vi "Collision Detection top level.vi"(0 "Model rotation (degrees)":sgl, 1 "Model rotation axis (unit vector)":sgl[](array[numeric])=[0.0, 0.0, 1.0], 3 "Model rotation axis coordinates (absolute, mm)":sgl[](array[numeric])=[0.0, 0.0, 0.0], 4 "Collision mode":T1=enum."Traverse - All", 5 "Get minimum separation within look-out sphere":bool, 6 "Traverse position (absolute, mm)":sgl[](array[numeric])=[0.0, 0.0, 0.0], 7 "3D graphics output":bool, 9 "Visualisation only (no collision detection)":bool, 10 "Traverse name":string="EnFlo_Trav1", 11 "Extrusion mode":bool, 12 "Rig geometry directory path":path=path "C:/EnFlo_Data_Local/Preferences/Rig_Setups/EnFlo_Tunnel/All_Users/Collision_detection", 13 "Traverse extruded position":sgl[](array[numeric])=[0.0, 0.0, 0.0]) -> (14 "Collision":bool, 15 "Collision point(s)":sgl[][](array[numeric]), 16 "Traverse collision part":cluster{"X":bool, "XY":bool, "XYZ":bool}, 17 "Minimum separation":sgl, 18 "Minimum separation vector (from trav.)":sgl[](array[numeric]), 19 "Error out":errorcluster)   [LabVIEW 2016]
uses:
  Collision Mode.ctl
  Typedefs/Triangle.ctl
  <vilib>/Utility/miscctls.llb/LVRGBAColorTypeDef.ctl
  Convex Hull/Subroutines/Coincident points test.vi
  Subroutines/Cross product 3D.vi
  Subroutines/Unit vector.vi
  Collision Detection global.vi
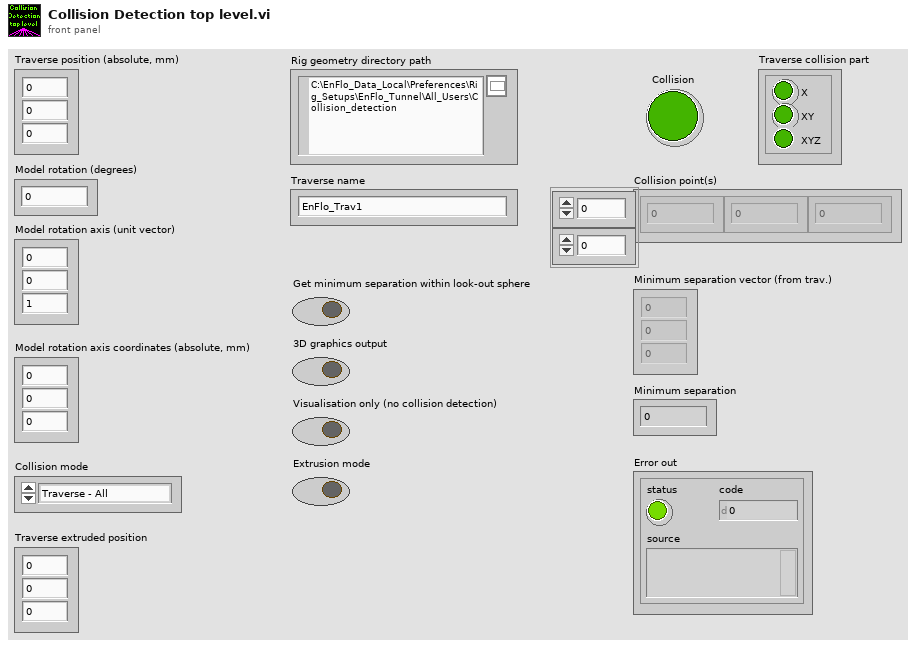
[diagram p1: front panel]
types:
  T1 = typedef "Collision Mode.ctl" = enum16{"Traverse - Tunnel", "Traverse - Model", "Traverse - Fixed objects", "Traverse - Traverse", "Traverse - All"}
  T2 = typedef "Traverse active parts.ctl" = enum16{"XYZ", "XY and XYZ", "X and XY and XYZ"}
  T3 = cluster{"Red":sgl, "Green":sgl, "Blue":sgl, "Alpha":sgl}
  T4 = typedef "LVRGBAColorTypeDef.ctl" = cluster{"Red":sgl, "Green":sgl, "Blue":sgl, "Alpha":sgl}
  T5 = typedef "TreeNodeBox.ctl" = cluster{"Face 0":T6, "Face 1":T6, "Face 2":T6, "Face 3":T6, "Face 4":T6, "Face 5":T6, "Level":i32, "Pmax":sgl[], "Pmin":sgl[], "Parent":i32, "Child 1":i32, "Child 2":i32, "Child 3":i32, "Child 4":i32, "Child 5":i32, "Child 6":i32, "Child 7":i32, "Child 8":i32, "Triangles":i32[], "is leaf node":bool}
  T6 = typedef "Quad.ctl" = cluster{"V0":sgl[], "V1":sgl[], "V2":sgl[], "V3":sgl[], "E0":sgl[], "E1":sgl[], "E2":sgl[], "E3":sgl[], "n^":sgl[], "Plane":T7}
  T7 = typedef "Quadplane enum.ctl" = enum8{"XY", "XZ", "YZ", "-XY", "-XZ", "-YZ"}
  T8 = typedef "Triangle.ctl" = cluster{"V0":sgl[], "V1":sgl[], "V2":sgl[], "E0":sgl[], "E1":sgl[], "E2":sgl[], "n^":sgl[], "nE0^":sgl[], "nE1^":sgl[], "nE2^":sgl[]}
  T9 = typedef "Sphere.ctl" = cluster{"Centre":sgl[], "Radius":sgl}
  T10 = typedef "Triangle, indexed.ctl" = cluster{"V0":sgl[], "V1":sgl[], "V2":sgl[], "n^":sgl[], "i0":i32, "i1":i32, "i2":i32}
  T11 = enum16{"Inherit Value", "Points", "Wireframe", "Polygons"}
  T12 = typedef "LV3DPointTypeDef.ctl" = cluster{"X":sgl, "Y":sgl, "Z":sgl}
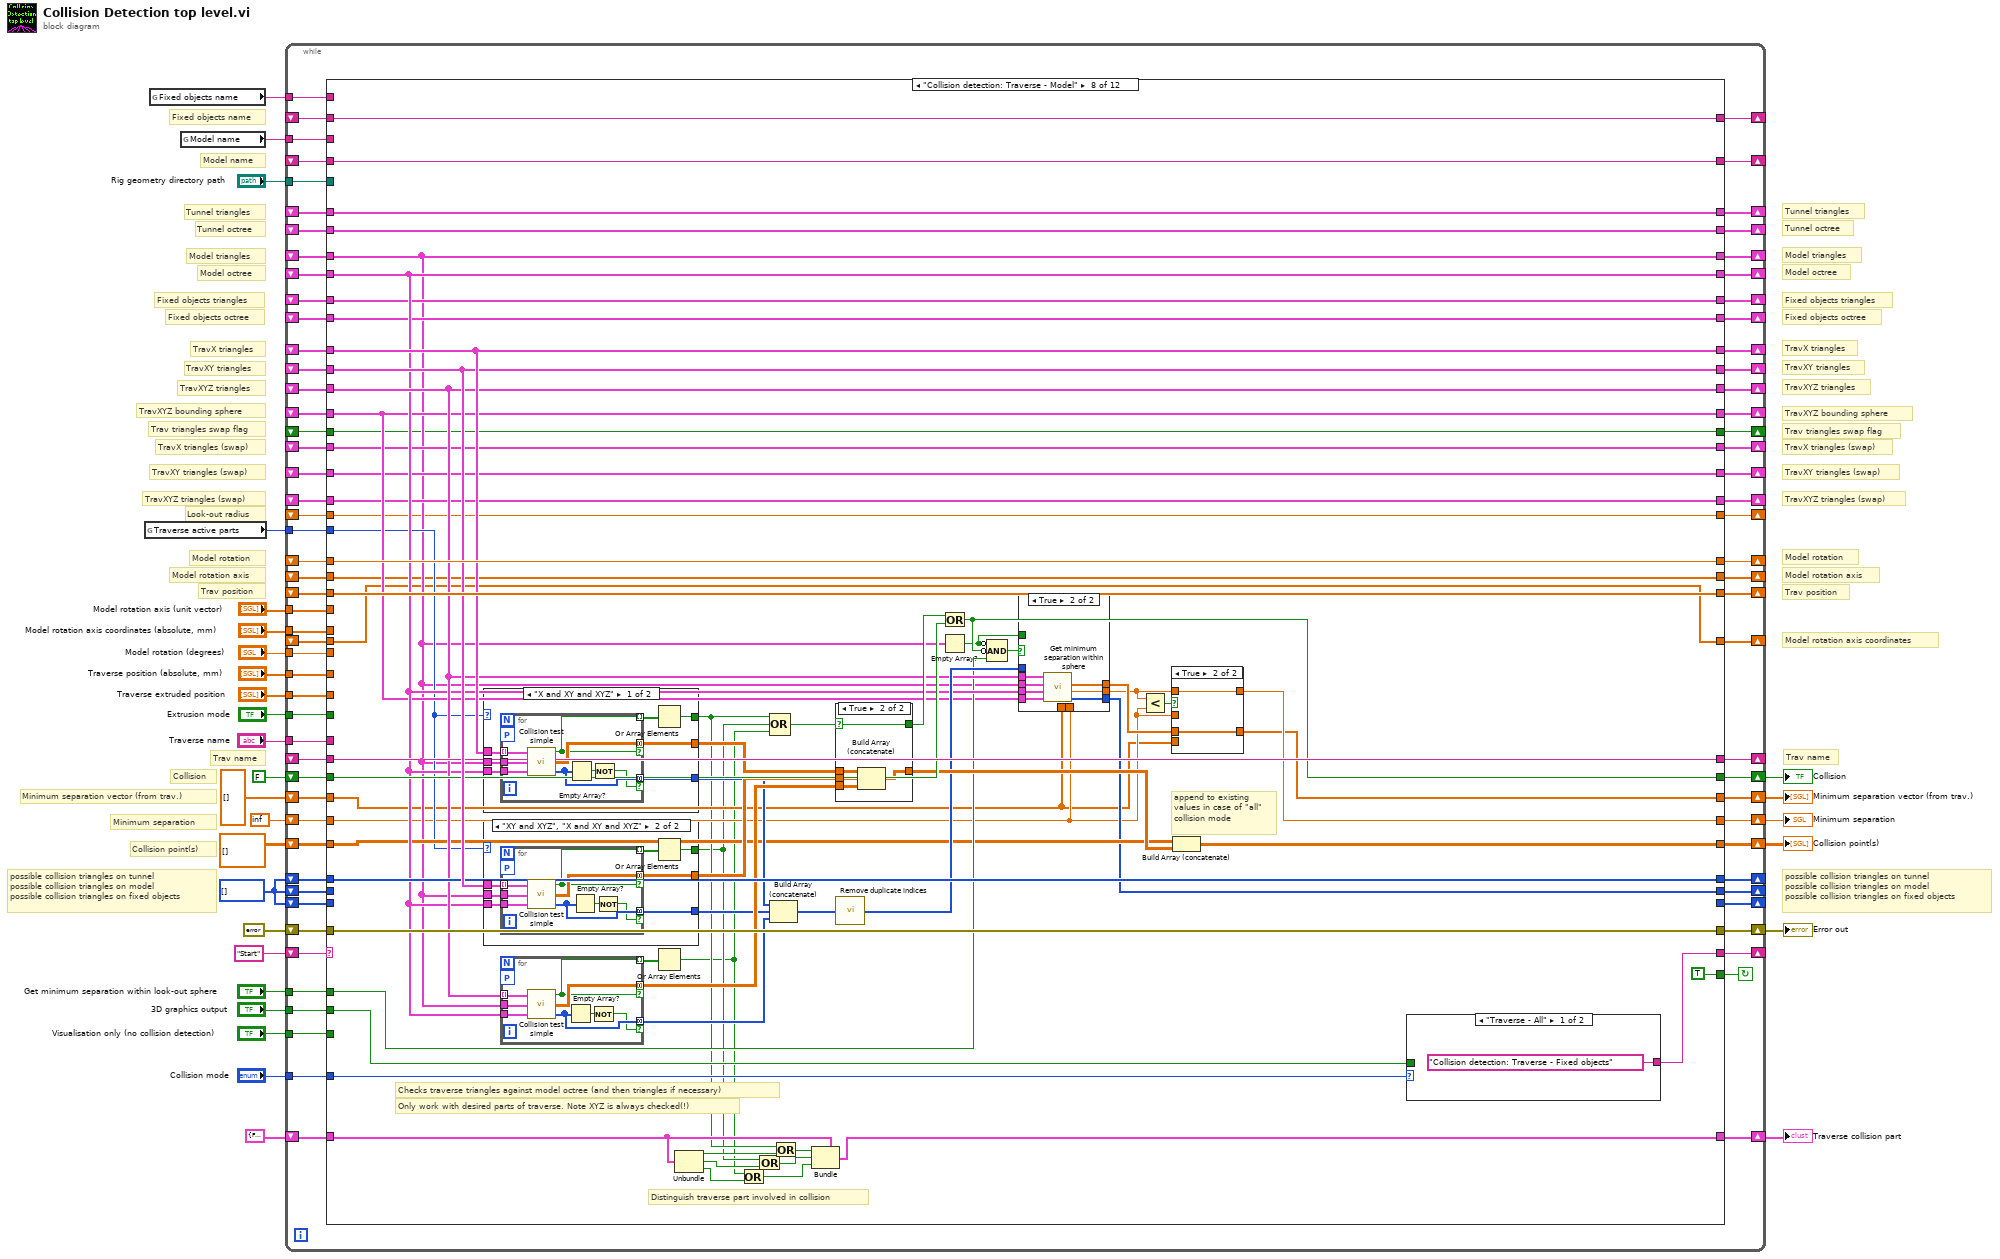
[diagram p0: block diagram]
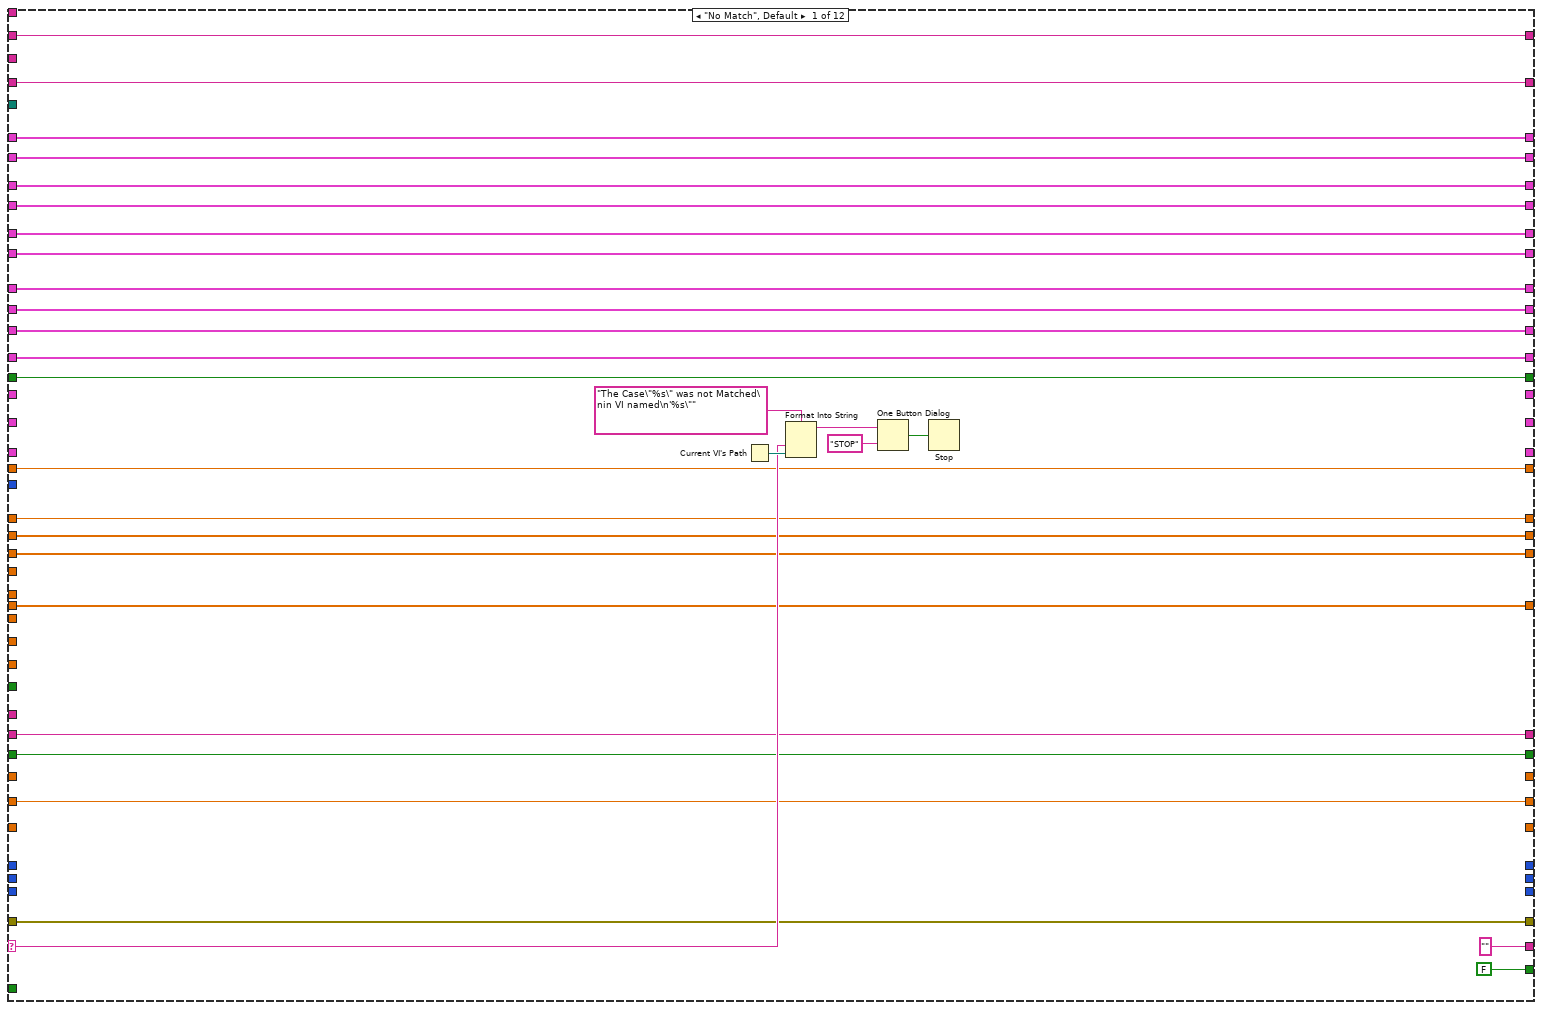
[diagram p2: hidden frame]
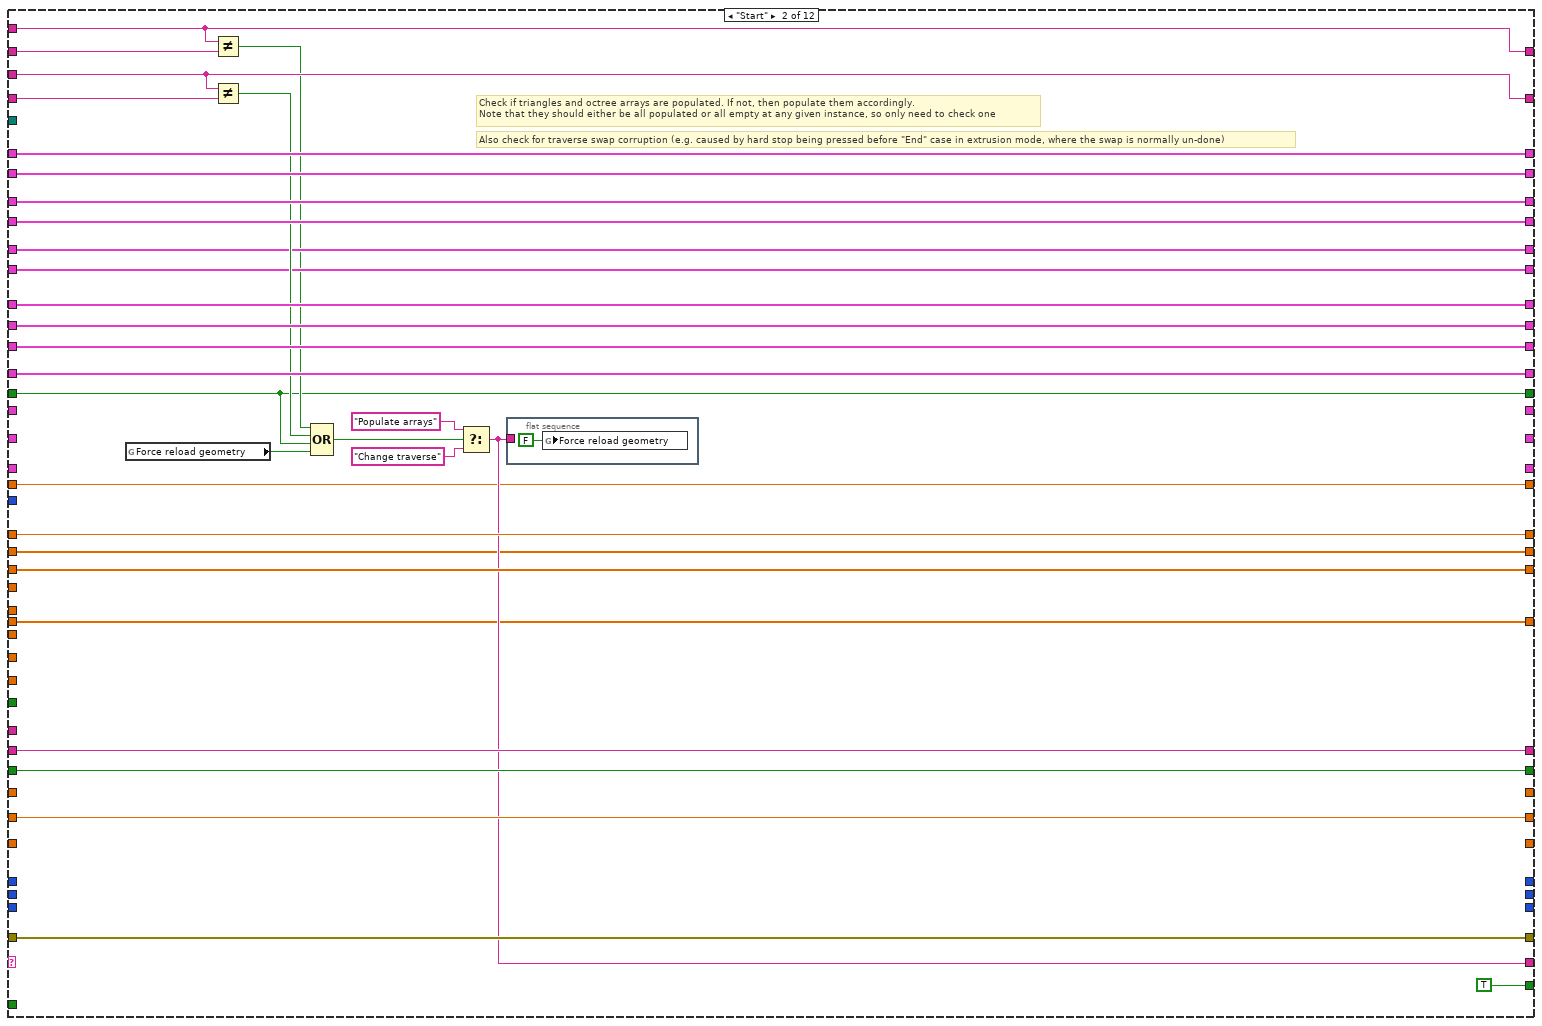
[diagram p3: hidden frame]
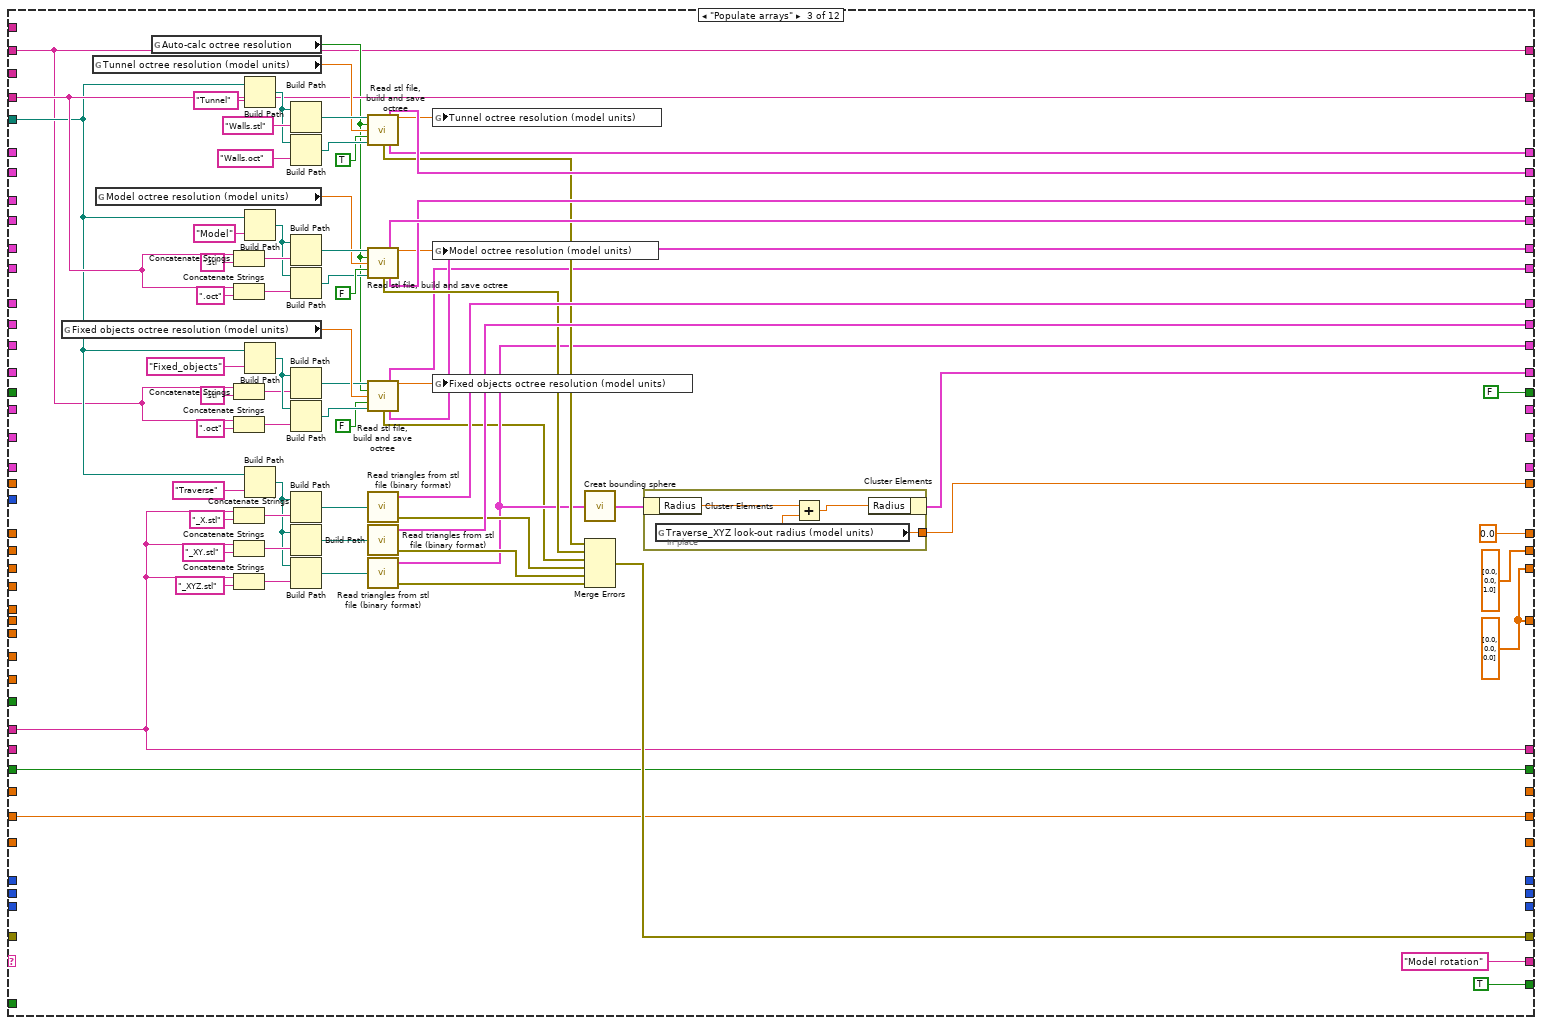
[diagram p4: hidden frame]
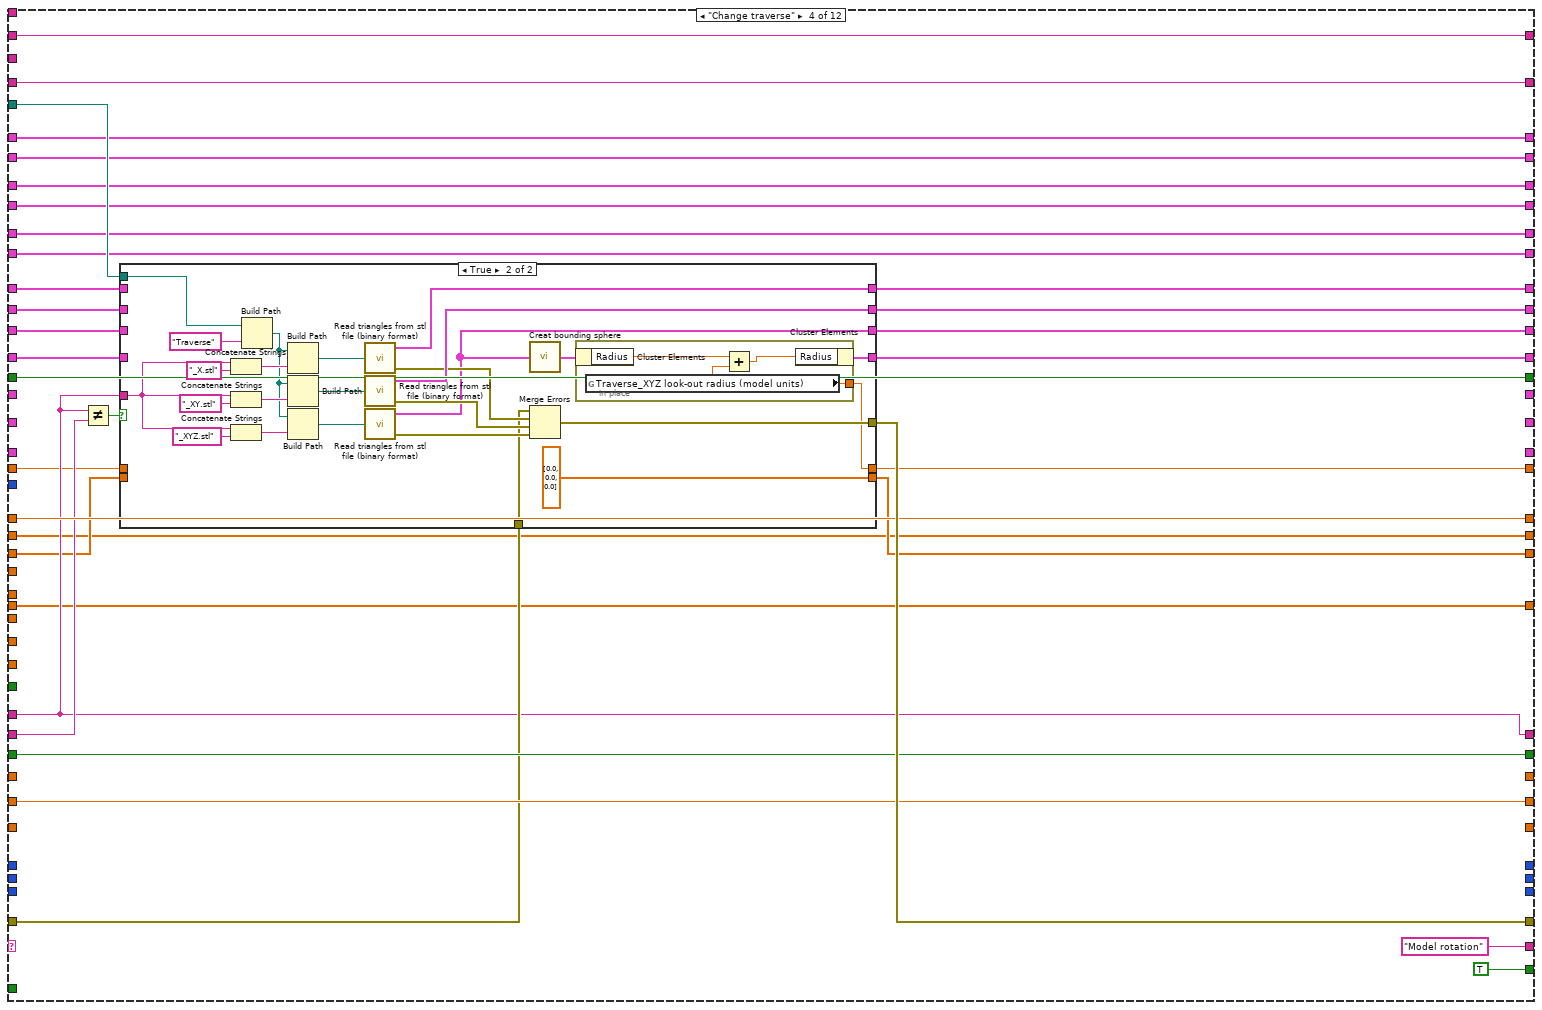
[diagram p5: hidden frame]
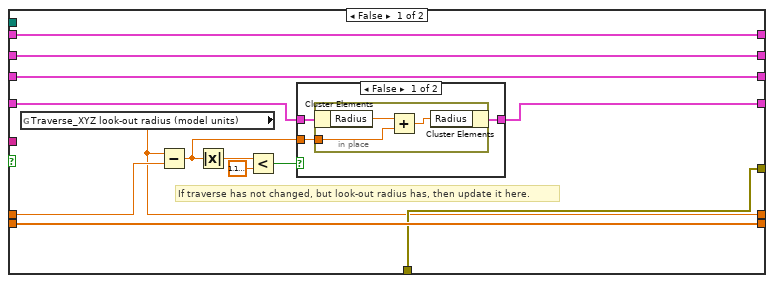
[diagram p6: hidden frame]
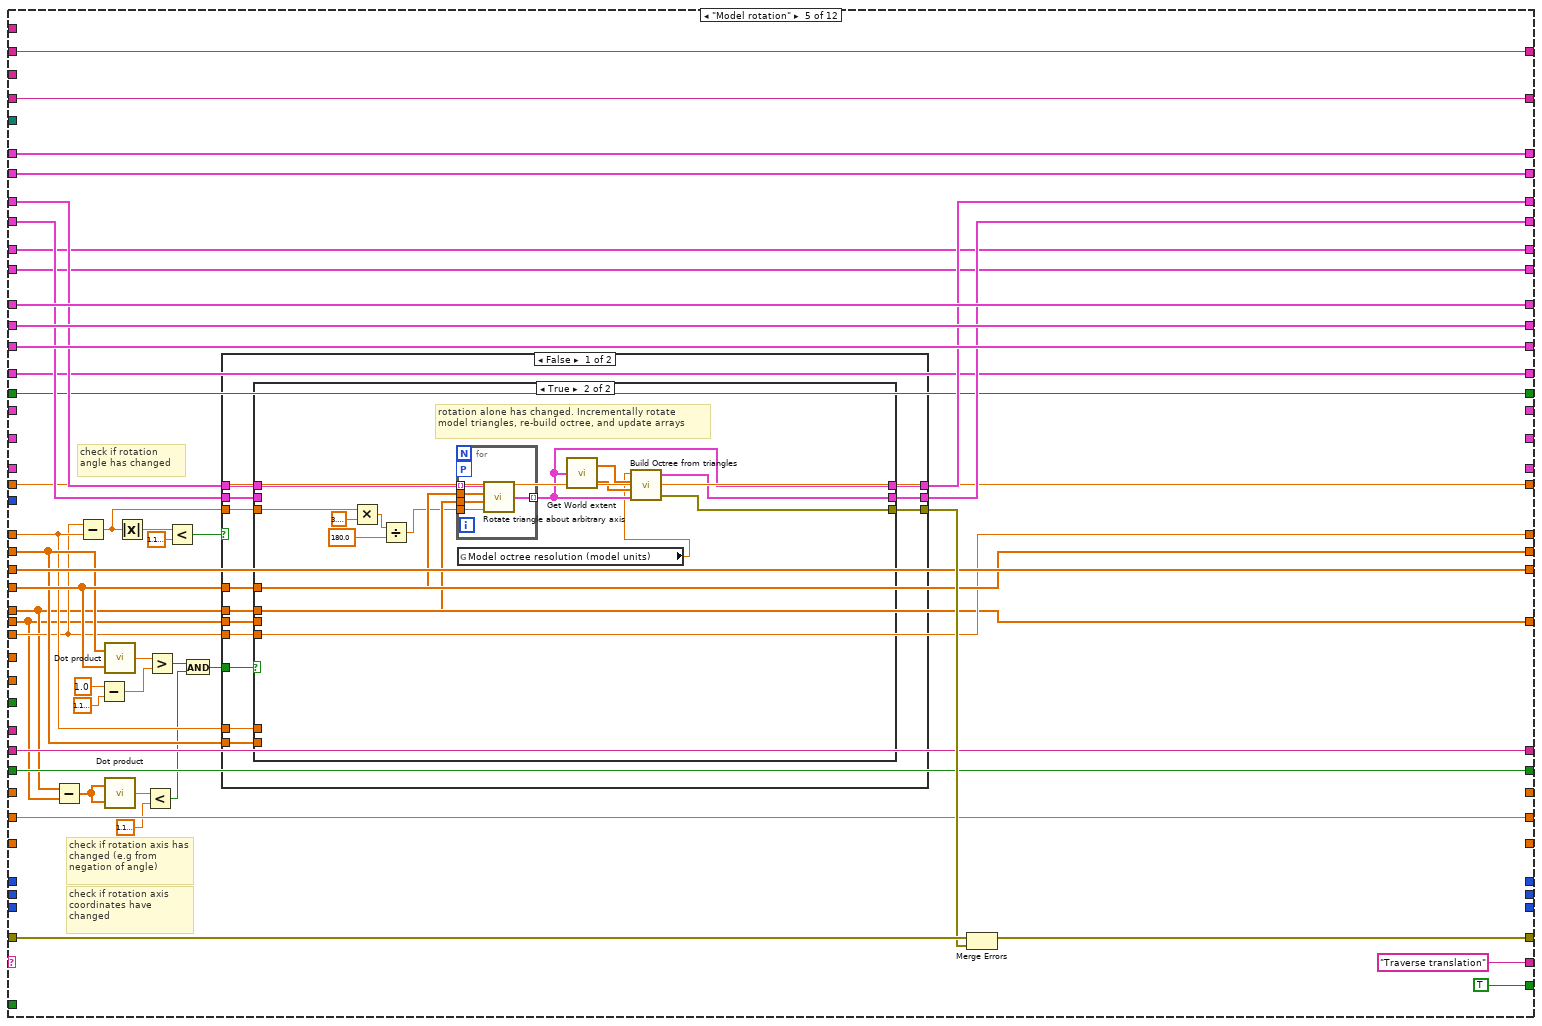
[diagram p8: hidden frame]
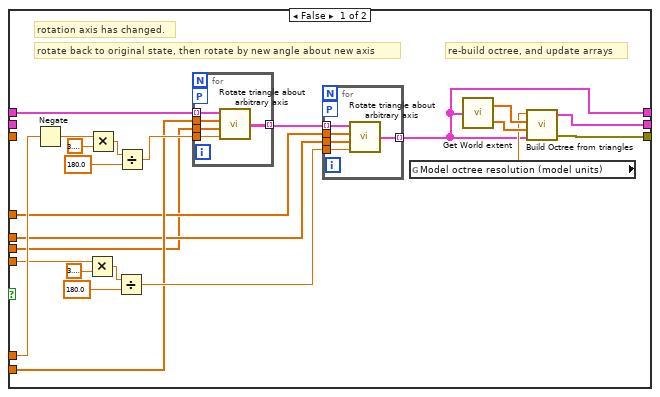
[diagram p9: hidden frame]
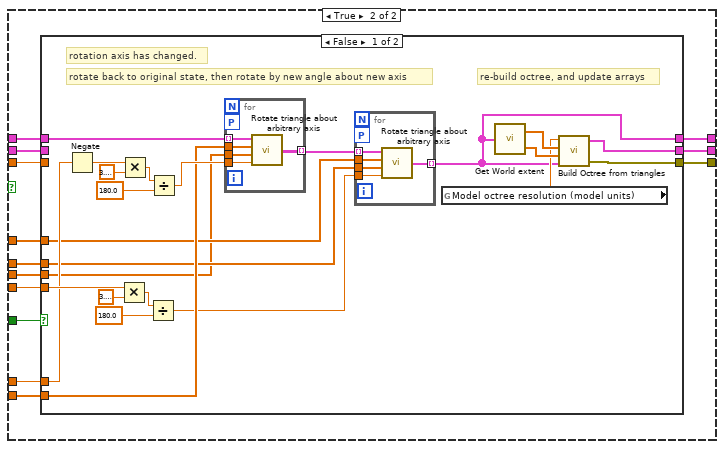
[diagram p10: hidden frame]
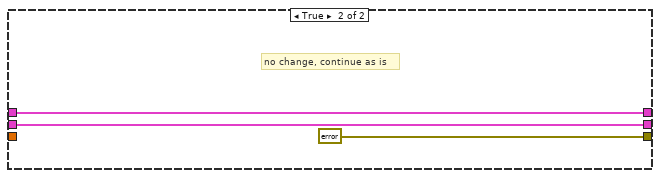
[diagram p11: hidden frame]
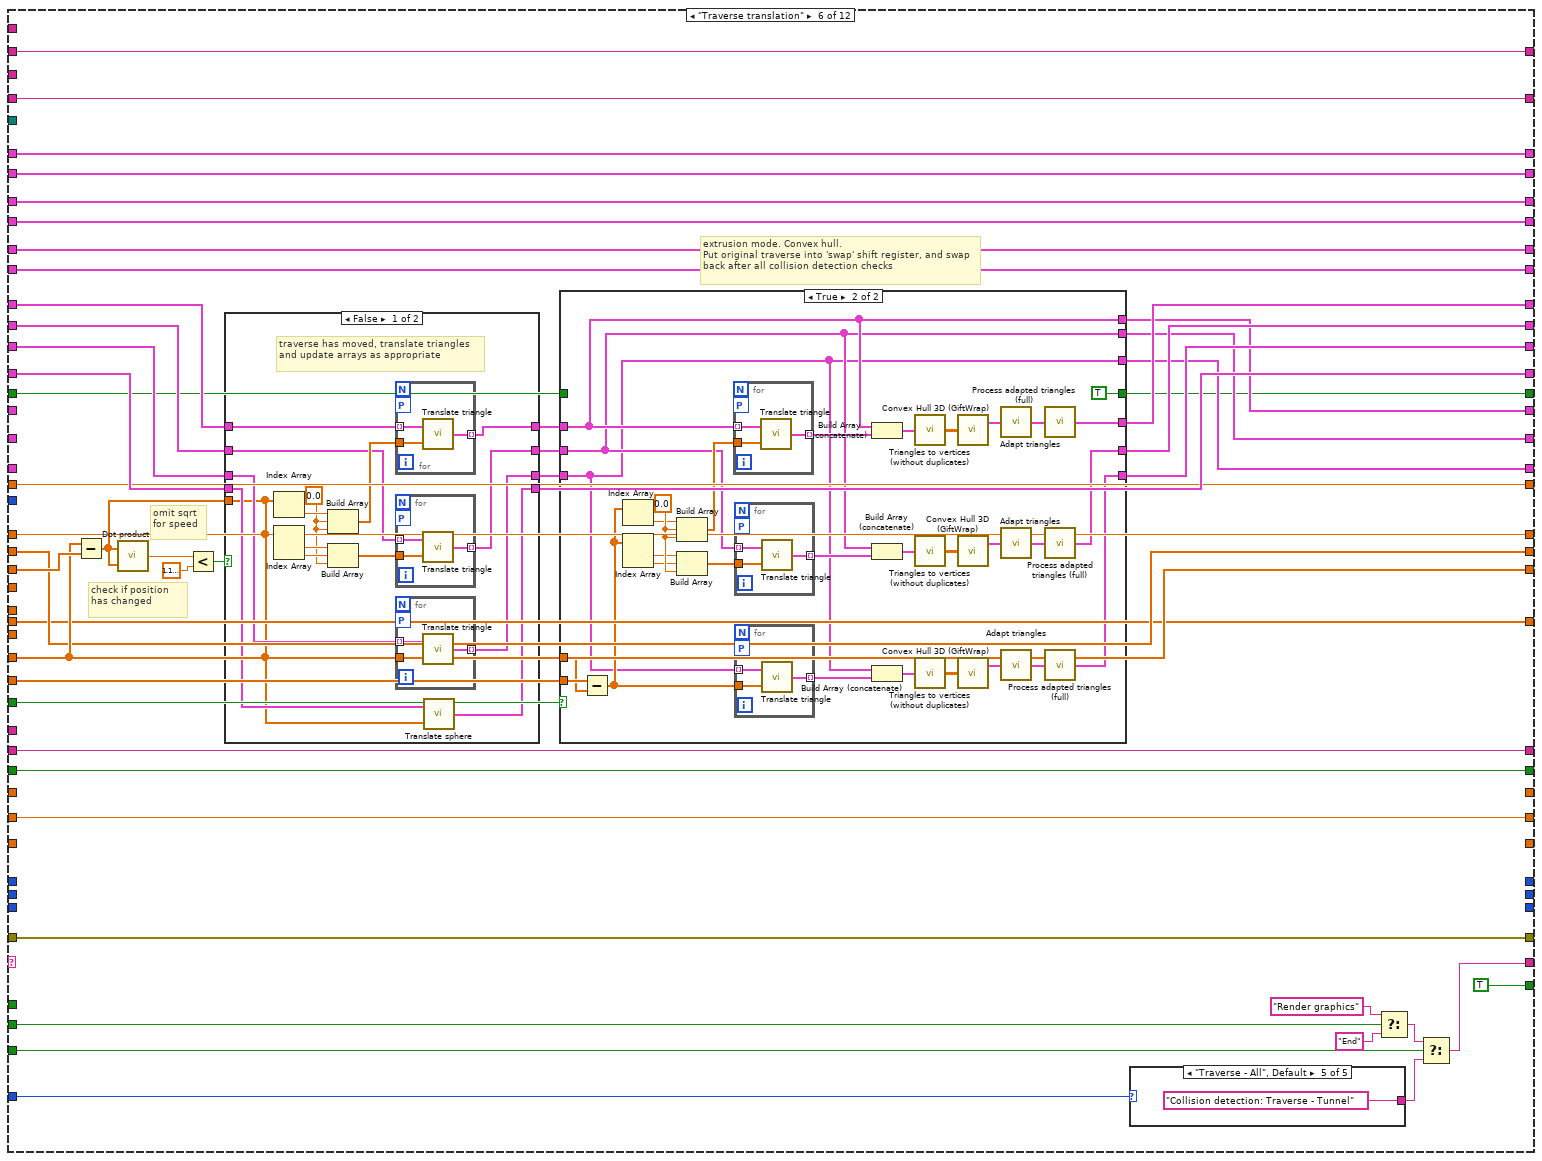
[diagram p12: hidden frame]
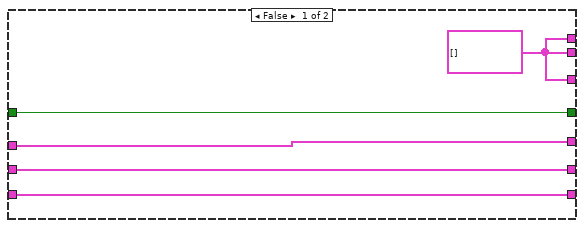
[diagram p13: hidden frame]
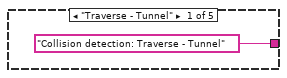
[diagram p14: hidden frame]
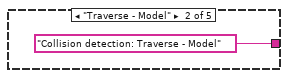
[diagram p15: hidden frame]
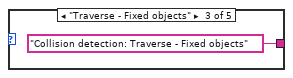
[diagram p16: hidden frame]
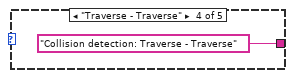
[diagram p17: hidden frame]
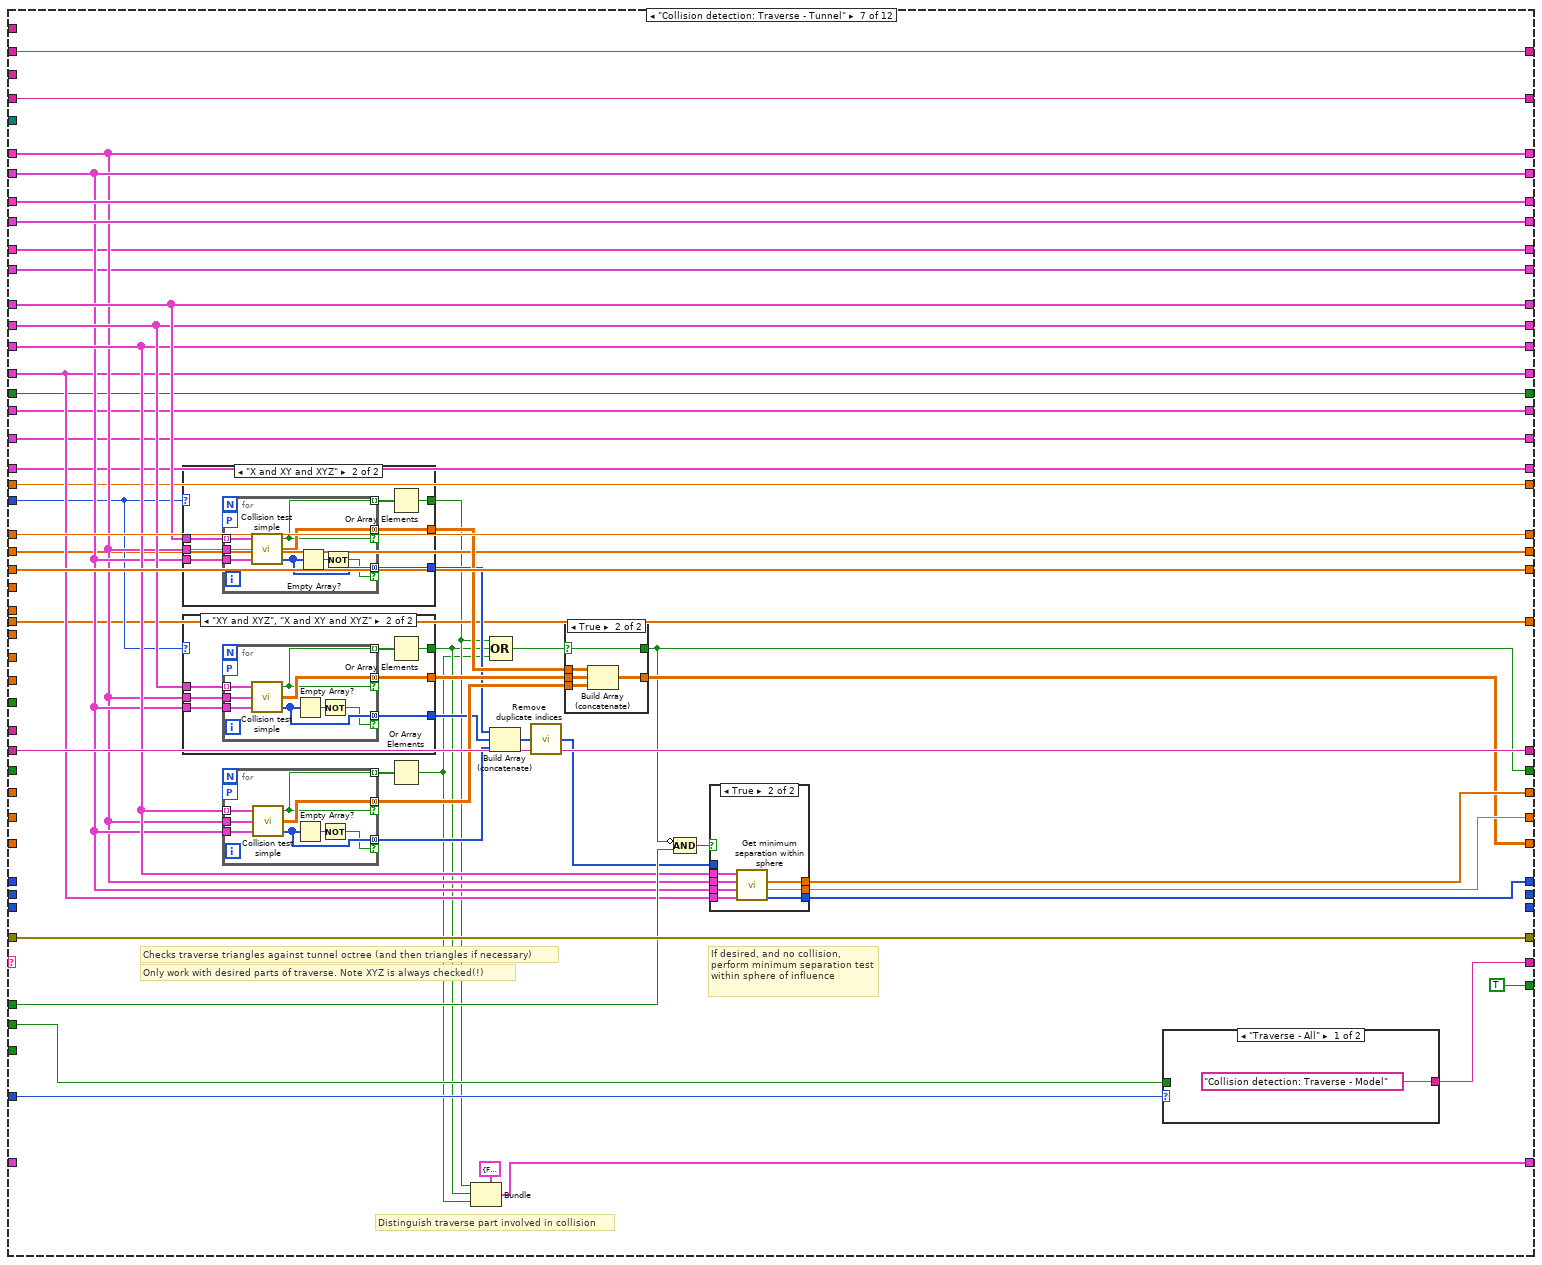
[diagram p19: hidden frame]
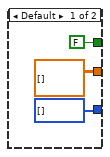
[diagram p20: hidden frame]
diagram:
  w3 = i32[] [] ("I32 array without duplicates")
  # "Look-out radius"
  # "Trav triangles swap flag"
  # "Trav triangles swap flag"
  # "Model rotation axis coordinates"
  # "Model rotation axis"
  # "Model rotation axis"
  # "Fixed objects octree"
  # "Fixed objects triangles"
  # "possible collision triangles on tunnel\npossible collision triangles on model\npossible collision triangles on fixed objects"
  # "Fixed objects name"
  # "Fixed objects octree"
  # "Fixed objects triangles"
  # "Model name"
  # "TravXYZ triangles (swap)"
  # "TravXY triangles (swap)"
  # "TravX triangles (swap)"
  # "TravXYZ triangles (swap)"
  # "TravXY triangles (swap)"
  # "TravX triangles (swap)"
  # "TravXYZ bounding sphere"
  # "TravXYZ bounding sphere"
  # "Trav name"
  # "Collision"
  # "Minimum separation vector (from trav.)"
  # "Minimum separation"
  # "Collision point(s)"
  # "Trav name"
  # "possible collision triangles on tunnel\npossible collision triangles on model\npossible collision triangles on fixed objects"
  # "Model rotation"
  # "Trav position"
  # "TravXYZ triangles"
  # "TravXY triangles"
  # "TravX triangles"
  # "Model octree"
  # "Model triangles"
  # "Tunnel octree"
  # "Tunnel triangles"
  # "Model rotation"
  # "Trav position"
  # "TravXYZ triangles"
  # "TravXY triangles"
  # "TravX triangles"
  # "Model octree"
  # "Model triangles"
  # "Tunnel octree"
  # "Tunnel triangles"
  n1 = global read "Collision Detection global.vi" "Traverse active parts"() -> (w7:T2)
  n2 = global read "Collision Detection global.vi" "Fixed objects name"() -> (w4:string)
  n3 = global read "Collision Detection global.vi" "Model name"() -> (w6:string)
  n4 = while {
    shift-right: [w91] -> _
    shift-left: "Start" -> [w109]
    shift-right: [w98] -> _
    shift-left: _ -> [w108]
    shift-right: [w97] -> _
    shift-left: _ -> [w107]
    shift-right: [w96] -> _
    shift-left: _ -> [w106]
    shift-right: [w95] -> _
    shift-left: _ -> [w105]
    shift-right: [w94] -> _
    shift-left: _ -> [w104]
    shift-right: [w93] -> _
    shift-left: _ -> [w103]
    shift-right: [w92] -> _
    shift-left: _ -> [w81]
    shift-right: [w85] -> _
    shift-left: _ -> [w101]
    shift-right: [w84] -> _
    shift-left: _ -> [w102]
    tunnel: "Traverse position (absolute, mm)" -> [w99]
    tunnel: "Model rotation (degrees)" -> [w100]
    tunnel: "Rig geometry directory path" -> [w89]
    shift-right: [w87] -> w16
    shift-left: errorcluster {"status"=FALSE, "code"=0, "source"=""} ("error IO") -> [w86]
    tunnel: "Model rotation axis (unit vector)" -> [w83]
    tunnel: "Model rotation axis coordinates (absolute, mm)" -> [w82]
    tunnel: "Get minimum separation within look-out sphere" -> [w80]
    tunnel: "Visualisation only (no collision detection)" -> [w79]
    tunnel: "3D graphics output" -> [w78]
    shift-right: [w74] -> _
    shift-left: w3 -> [w72]
    shift-right: [w73] -> _
    shift-left: w3 -> [w71]
    shift-right: [w75] -> w18
    shift-left: sgl[] [] -> [w70]
    shift-right: [w76] -> w19
    shift-left: sgl inf -> [w69]
    shift-right: [w63] -> w17
    shift-left: sgl[][] [] -> [w68]
    shift-right: [w77] -> w20
    shift-left: FALSE -> [w67]
    shift-right: [w66] -> _
    shift-left: _ -> [w88]
    tunnel: "Traverse name" -> [w65]
    tunnel: "Collision mode" -> [w64]
    shift-right: [w61] -> _
    shift-left: _ -> [w62]
    tunnel: "Traverse extruded position" -> [w60]
    tunnel: "Extrusion mode" -> [w59]
    shift-right: [w58] -> _
    shift-left: _ -> [w55]
    shift-right: [w57] -> _
    shift-left: _ -> [w54]
    shift-right: [w56] -> _
    shift-left: _ -> [w53]
    tunnel: w7 -> [w52]
    tunnel: w6 -> [w51]
    shift-right: [w49] -> _
    shift-left: _ -> [w50]
    shift-right: [w46] -> _
    shift-left: _ -> [w48]
    shift-right: [w45] -> _
    shift-left: _ -> [w47]
    tunnel: w4 -> [w44]
    shift-right: [w42] -> _
    shift-left: _ -> [w43]
    shift-right: [w40] -> _
    shift-left: w3 -> [w41]
    shift-right: [w38] -> _
    shift-left: _ -> [w39]
    shift-right: [w36] -> _
    shift-left: _ -> [w37]
    shift-right: [w34] -> w2
    shift-left: cluster{"X":bool, "XY":bool, "XYZ":bool} {"X"=FALSE, "XY"=FALSE, "XYZ"=FALSE} ("Traverse collision part") -> [w35]
    shift-right: [w32] -> _
    shift-left: _ -> [w33]
    shift-right: [w30] -> _
    shift-left: _ -> [w31]
    stop <- w90 continue-if-true
    n5 = case shown="\"Collision detection: Traverse - Model\"" w109 {
      selector: w109 -> [w134 _ _ _ _ _ _ _ _ _ _ _]
      tunnel: w108 -> [w130 w161 _ w273 w374 w532 w638 w795 w939 w1047 w1129 w1285]
      tunnel: w107 -> [w129 w162 _ w272 w373 w531 w639 w794 w938 w1046 w1125 w1284]
      tunnel: w106 -> [w128 w153 _ w271 w369 w530 w661 w752 w910 w1043 w1087 w1283]
      tunnel: w105 -> [w127 w163 _ w270 w364 w529 w660 w766 w909 w1042 w1124 w1282]
      tunnel: w104 -> [w126 w164 _ w266 w372 w536 w663 w796 w940 w1048 w1128 w1269]
      tunnel: w103 -> [w125 w165 _ w265 w371 w535 w662 w793 w937 w1045 w1127 w1270]
      tunnel: w81 -> [w124 w166 _ w264 w370 w534 w640 w767 w911 w1044 w1126 w1271]
      tunnel: w102 -> [w122 w159 _ w262 w356 w539 w666 w799 w943 w1055 w1133 w1287]
      tunnel: w101 -> [w123 w160 _ w276 w344 w516 w667 w800 w944 w1056 w1134 w1286]
      tunnel: w100 -> [_ _ _ _ w343 _ _ _ _ _ _ _]
      tunnel: w99 -> [_ _ _ _ _ w509 _ _ _ _ _ _]
      tunnel: [w130 w161 w241 w273 w374 w532 w638 w795 w939 w1047 w1129 w1285] -> w98
      tunnel: [w129 w162 w242 w272 w373 w531 w639 w794 w938 w1046 w1125 w1284] -> w97
      tunnel: [w128 w153 w243 w271 w366 w530 w661 w752 w910 w1043 w1087 w1283] -> w96
      tunnel: [w127 w163 w244 w270 w365 w529 w660 w766 w909 w1042 w1124 w1282] -> w95
      tunnel: [w126 w164 w245 w281 w372 w505 w663 w796 w940 w1048 w1128 w1274] -> w94
      tunnel: [w125 w165 w246 w282 w371 w504 w662 w793 w937 w1045 w1127 w1273] -> w93
      tunnel: [w124 w166 w199 w283 w370 w503 w640 w767 w911 w1044 w1126 w1272] -> w92
      tunnel: [w123 w160 sgl 0.0 ("Numeric") w276 w343 w516 w667 w800 w944 w1056 w1134 w1286] -> w85
      tunnel: [w122 w159 w175 w261 w356 w509 w666 w799 w943 w1055 w1133 w1287] -> w84
      tunnel: w89 -> [_ _ w181 w280 _ _ _ _ _ _ _ _]
      tunnel: ["" w155 "Model rotation" "Model rotation" "Traverse translation" w525 w653 w785 w929 w1051 "End" "" ("f")] -> w91
      tunnel: [FALSE TRUE TRUE TRUE TRUE TRUE TRUE TRUE TRUE TRUE TRUE FALSE] -> w90
      tunnel: w88 -> [w119 w156 _ w268 w357 w518 w657 w792 w936 w1041 w1094 w1280]
      tunnel: [w131 w167 w240 w279 w363 w527 w664 w797 w941 w1049 w1112 w1288] -> w87
      tunnel: w86 -> [w131 w167 _ w269 w362 w527 w664 w797 w941 w1049 w1113 w1288]
      tunnel: w83 -> [_ _ _ _ w350 _ _ _ _ _ _ _]
      tunnel: w82 -> [_ _ _ _ w337 _ _ _ _ _ _ _]
      tunnel: w80 -> [_ _ _ _ _ _ w644 w765 w908 _ _ w1255]
      tunnel: w79 -> [_ _ _ _ _ w526 _ _ _ _ _ _]
      tunnel: w78 -> [_ _ _ _ _ w524 w654 w784 w928 w1052 _ _]
      tunnel: [w120 w157 w205 w274 w358 w519 w645 w768 w912 w1040 w1130 w1281] -> w77
      tunnel: [w121 w158 w206 w275 w359 w520 w659 w788 w932 w1038 w1131 w1256] -> w76
      tunnel: [_ _ _ _ _ _ w658 w787 w931 w1039 w1132 w1258] -> w75
      tunnel: [_ _ _ _ _ _ w656 w790 w934 w1035 w1062 w1264] -> w63
      tunnel: [_ _ _ _ _ _ w641 w791 w935 w1037 _ _] -> w74
      tunnel: [_ _ _ _ _ _ _ _ w897 w1036 _ _] -> w73
      tunnel: w72 -> [_ _ _ _ _ _ _ w791 w935 w1037 w1104 _]
      tunnel: w71 -> [_ _ _ _ _ _ _ _ _ w1036 w1063 _]
      tunnel: w70 -> [_ _ _ _ _ _ _ w750 w894 w1039 w1132 w1258]
      tunnel: w69 -> [w121 w158 w206 w275 w359 w520 _ w751 w893 w1038 w1131 w1257]
      tunnel: w68 -> [_ _ _ _ _ _ _ w760 w903 w1035 w1062 w1264]
      tunnel: w67 -> [w120 w157 w205 w274 w358 w519 _ w782 w926 w1040 w1130 w1281]
      tunnel: [w119 w156 w204 w263 w357 w518 w657 w792 w936 w1041 w1094 w1280] -> w66
      tunnel: w65 -> [_ _ w204 w263 _ _ _ _ _ _ _ _]
      tunnel: w64 -> [_ _ _ _ _ w515 w655 w786 w930 _ _ _]
      tunnel: w62 -> [w118 w154 _ w259 w355 w513 w637 w764 w907 w1034 w1081 w1279]
      tunnel: [w118 w154 w197 w260 w355 w512 w637 w764 w907 w1034 w1081 w1279] -> w61
      tunnel: w60 -> [_ _ _ _ _ w510 _ _ _ _ _ _]
      tunnel: w59 -> [_ _ _ _ _ w511 _ _ _ _ _ w1278]
      tunnel: [_ _ _ _ _ w500 w636 w763 w906 w1033 w1080 _] -> w58
      tunnel: [_ _ _ _ _ w501 w635 w762 w905 w1032 w1079 _] -> w57
      tunnel: [_ _ _ _ _ w502 w634 w761 w904 w1031 w1078 _] -> w56
      tunnel: w55 -> [_ _ _ _ _ _ w636 w763 w906 w1033 w1080 w1277]
      tunnel: w54 -> [_ _ _ _ _ _ w635 w762 w905 w1032 w1079 w1276]
      tunnel: w53 -> [_ _ _ _ _ _ w634 w761 w904 w1031 w1078 w1275]
      tunnel: w52 -> [_ _ _ _ _ _ w632 w758 w901 _ _ _]
      tunnel: w51 -> [_ w152 _ _ _ _ _ _ _ _ _ _]
      tunnel: w50 -> [w117 w151 w194 w258 w354 w499 w630 w757 w900 w1030 w1076 w1268]
      tunnel: [w117 w152 w194 w258 w354 w499 w630 w757 w900 w1030 w1076 w1268] -> w49
      tunnel: w48 -> [w116 w149 _ w256 w351 w497 w628 w755 w895 w1028 w1071 w1266]
      tunnel: w47 -> [w115 w148 _ w255 w352 w496 w627 w754 w898 w1027 w1074 w1265]
      tunnel: [w116 w149 w178 w256 w351 w497 w628 w755 w895 w1028 w1071 w1266] -> w46
      tunnel: [w115 w148 w177 w255 w352 w496 w627 w754 w898 w1027 w1074 w1265] -> w45
      tunnel: w44 -> [_ w145 _ _ _ _ _ _ _ _ _ _]
      tunnel: w43 -> [w114 w147 w180 w257 w353 w498 w629 w756 w899 w1029 w1075 w1267]
      tunnel: [w114 w145 w180 w257 w353 w498 w629 w756 w899 w1029 w1075 w1267] -> w42
      tunnel: w41 -> [_ _ _ _ _ _ _ _ w896 w1026 w1064 _]
      tunnel: [_ _ _ _ _ _ _ w753 w896 w1026 _ _] -> w40
      tunnel: w39 -> [w113 w144 _ w254 w345 w495 w626 w748 w891 w1025 w1061 w1263]
      tunnel: [w113 w144 sgl[] [0.0, 0.0, 1.0] ("Traverse position (absolute, mm)") w254 w350 w495 w626 w748 w891 w1025 w1061 w1263] -> w38
      tunnel: w37 -> [w112 w143 _ w253 w334 w494 w625 w747 w890 w1024 w1060 w1262]
      tunnel: [w112 w143 w175 w253 w337 w494 w625 w747 w890 w1024 w1060 w1262] -> w36
      tunnel: w35 -> [_ _ _ _ _ _ _ w746 w883 w1023 w1059 w1261]
      tunnel: [_ _ _ _ _ _ w621 w736 w882 w1023 w1059 w1261] -> w34
      tunnel: w33 -> [w111 w141 _ w252 w333 w492 w619 w735 w878 w1022 w1058 w1259]
      tunnel: [w111 w141 FALSE w252 w333 w493 w619 w735 w878 w1022 w1058 w1260] -> w32
      tunnel: w31 -> [w110 w140 _ w251 w332 w491 w618 w734 w877 w1021 w1057 w1254]
      tunnel: [w110 w140 w173 w250 w332 w491 w618 w734 w877 w1021 w1057 w1254] -> w30
      frame "No Match", Default {
        n6 = Current VI's Path() -> (path=w135:path)
        n7 = Format Into String(format string="The Case\"%s\" was not Matched\nin VI named\n'%s\"" ("Format String"), w134, w135) -> (resulting string=w138:string)  [unwired: 2 in, 1 out]
        n8 = One Button Dialog(message=w138, button name ("OK")="STOP") -> (true=w136:bool)
        n9 = Stop(stop? (T)=w136) -> ()
      }
      frame "Start" {
        # "Also check for traverse swap corruption (e.g. caused by hard stop being pressed before \"End\" case in extrusion mode, where the swap is normally un-done)"
        # "Check if triangles and octree arrays are populated. If not, then populate them accordingly.\nNote that they should either be all populated or all empty at any given instance, so only need to check one"
        n10 = global read "Collision Detection global.vi" "Force reload geometry"() -> (w142:bool)
        n11 = Not Equal?(x=w145, y=w147) -> (x != y?=w146:bool)
        n12 = Not Equal?(x=w152, y=w151) -> (x != y?=w150:bool)
        n13 = Compound Arithmetic op=OR(w146, w150, w141, w142) -> (w171:bool)
        n14 = Select(t="Populate arrays", s=w171, f="Change traverse") -> (s? t:f=w155:string)
        n15 = flat-sequence {
          tunnel: w155 -> [_]
          frame #0 {
            n16 = global write "Collision Detection global.vi" "Force reload geometry"(FALSE ("Force reload geometry")) -> ()
          }
        }
      }
      frame "Populate arrays" {
        w175 = sgl[] [0.0, 0.0, 0.0] ("Traverse position (absolute, mm)")
        n17 = global read "Collision Detection global.vi" "Fixed objects octree resolution (model units)"() -> (w192:sgl)
        n18 = global read "Collision Detection global.vi" "Tunnel octree resolution (model units)"() -> (w202:sgl)
        n19 = global read "Collision Detection global.vi" "Model octree resolution (model units)"() -> (w201:sgl)
        n20 = global read "Collision Detection global.vi" "Auto-calc octree resolution"() -> (w182:bool)
        n21 = Concatenate Strings(w194, ".stl" ("string")) -> (w229:string)
        n22 = Concatenate Strings(w194, ".oct" ("string")) -> (w228:string)
        n23 = Concatenate Strings(w180, ".stl" ("string")) -> (w186:string)
        n24 = Concatenate Strings(w180, ".oct" ("string")) -> (w187:string)
        n25 = Concatenate Strings(w204, "_X.stl" ("string")) -> (w223:string)
        n26 = Concatenate Strings(w204, "_XY.stl" ("string")) -> (w214:string)
        n27 = Concatenate Strings(w204, "_XYZ.stl" ("string")) -> (w212:string)
        n28 = Build Path(base path=w181, name or relative path="Tunnel") -> (appended path=w236:path)
        n29 = Build Path(base path=w181, name or relative path="Model") -> (appended path=w227:path)
        n30 = Build Path(base path=w181, name or relative path="Fixed_objects") -> (appended path=w188:path)
        n31 = Build Path(base path=w181, name or relative path="Traverse") -> (appended path=w203:path)
        n32 = Build Path(base path=w236, name or relative path="Walls.stl") -> (appended path=w237:path)
        n33 = Build Path(base path=w236, name or relative path="Walls.oct") -> (appended path=w234:path)
        n34 = Build Path(base path=w227, name or relative path=w229) -> (appended path=w225:path)
        n35 = Build Path(base path=w227, name or relative path=w228) -> (appended path=w224:path)
        n36 = Build Path(base path=w188, name or relative path=w186) -> (appended path=w190:path)
        n37 = Build Path(base path=w188, name or relative path=w187) -> (appended path=w191:path)
        n38 = Build Path(base path=w203, name or relative path=w223) -> (appended path=w220:path)
        n39 = Build Path(base path=w203, name or relative path=w214) -> (appended path=w216:path)
        n40 = Build Path(base path=w203, name or relative path=w212) -> (appended path=w210:path)
        n41 = call "Read stl file, build and save octree.vi"("STL file path (load)"=w237, "Auto resolution"=w182, "Specify resolution"=w202, "Invert model (interior region)"=TRUE, "Octree file path (save)"=w234) -> ("Octree node array"=w242:T5[], "Octree resolution"=w196:sgl, "Error out"=w219:errorcluster, "Triangles array"=w241:T8[])  [unwired: 3 in, 4 out]
        n42 = call "Read stl file, build and save octree.vi"("STL file path (load)"=w225, "Auto resolution"=w182, "Specify resolution"=w201, "Invert model (interior region)"=FALSE, "Octree file path (save)"=w224) -> ("Octree node array"=w244:T5[], "Octree resolution"=w195:sgl, "Error out"=w218:errorcluster, "Triangles array"=w243:T8[])  [unwired: 3 in, 4 out]
        n43 = call "Read stl file, build and save octree.vi"("STL file path (load)"=w190, "Auto resolution"=w182, "Specify resolution"=w192, "Invert model (interior region)"=FALSE, "Octree file path (save)"=w191) -> ("Octree node array"=w177:T5[], "Octree resolution"=w193:sgl, "Error out"=w179:errorcluster, "Triangles array"=w178:T8[])  [unwired: 3 in, 4 out]
        n44 = call "Read triangles from stl file (binary format).vi"("STL file path"=w220) -> ("Triangles array"=w245:T8[], "Error out"=w217:errorcluster)  [unwired: 1 out]
        n45 = call "Read triangles from stl file (binary format).vi"("STL file path"=w216) -> ("Triangles array"=w246:T8[], "Error out"=w213:errorcluster)  [unwired: 1 out]
        n46 = call "Read triangles from stl file (binary format).vi"("STL file path"=w210) -> ("Triangles array"=w199:T8[], "Error out"=w209:errorcluster)  [unwired: 1 out]
        n47 = global write "Collision Detection global.vi" "Tunnel octree resolution (model units)"(w196) -> ()
        n48 = global write "Collision Detection global.vi" "Model octree resolution (model units)"(w195) -> ()
        n49 = global write "Collision Detection global.vi" "Fixed objects octree resolution (model units)"(w193) -> ()
        n50 = call "Creat bounding sphere.vi"("Triangles"=w199) -> ("Bounding sphere"=w198:T9)
        n51 = Merge Errors(w219, w218, w179, w217, w213, w209) -> (w240:errorcluster)
        n52 = in-place {
          in-place-border: [w247] -> w173
          n53 = in-place-cluster #1(w198) -> ("Radius"=w249:sgl)
          n54 = global read "Collision Detection global.vi" "Traverse_XYZ look-out radius (model units)"() -> (w247:sgl)
          n55 = Add(x=w249, y=w247) -> (x+y=w248:sgl)
          n56 = in-place-cluster #1("Radius"=w248) -> (w197:T9)
        }
      }
      frame "Change traverse" {
        n57 = Not Equal?(x=w263, y=w268) -> (x != y?=w267:bool)
        n58 = case shown="True" w267 {
          tunnel: [w294 w307] -> w283
          tunnel: [w295 w328] -> w282
          tunnel: [w296 w327] -> w281
          tunnel: w280 -> [_ w326]
          tunnel: [w289 w325] -> w279
          tunnel: w263 -> [_ w309]
          tunnel: w269 -> [w289 w311]
          tunnel: w266 -> [w296 _]
          tunnel: w265 -> [w295 _]
          tunnel: w264 -> [w294 _]
          tunnel: w262 -> [w293 _]
          tunnel: [w293 sgl[] [0.0, 0.0, 0.0] ("Traverse position (absolute, mm)")] -> w261
          tunnel: [w287 w305] -> w260
          tunnel: w259 -> [w288 _]
          tunnel: w251 -> [w290 _]
          tunnel: [w284 w304] -> w250
          frame False {
            # "If traverse has not changed, but look-out radius has, then update it here."
            n59 = global read "Collision Detection global.vi" "Traverse_XYZ look-out radius (model units)"() -> (w284:sgl)
            n60 = Subtract(x=w284, y=w290) -> (x-y=w286:sgl)
            n61 = Absolute Value(x=w286) -> (abs(x)=w292:sgl)
            n62 = Less?(x=w292, y=sgl 1.1920929e-07) -> (x < y?=w285:bool)
            n63 = case shown="False" w285 {
              tunnel: w288 -> [w299 w303]
              tunnel: [w298 w303] -> w287
              tunnel: w286 -> [w297 _]
              frame False {
                n64 = in-place {
                  in-place-border: w297 -> [w300]
                  n65 = in-place-cluster #2(w299) -> ("Radius"=w302:sgl)
                  n66 = Add(x=w302, y=w300) -> (x+y=w301:sgl)
                  n67 = in-place-cluster #2("Radius"=w301) -> (w298:T9)
                }
              }
              frame True {
              }
            }
          }
          frame True {
            n68 = Concatenate Strings(w309, "_X.stl" ("string")) -> (w324:string)
            n69 = Concatenate Strings(w309, "_XY.stl" ("string")) -> (w317:string)
            n70 = Concatenate Strings(w309, "_XYZ.stl" ("string")) -> (w315:string)
            n71 = Build Path(base path=w326, name or relative path="Traverse") -> (appended path=w310:path)
            n72 = Build Path(base path=w310, name or relative path=w324) -> (appended path=w321:path)
            n73 = Build Path(base path=w310, name or relative path=w317) -> (appended path=w319:path)
            n74 = Build Path(base path=w310, name or relative path=w315) -> (appended path=w313:path)
            n75 = call "Read triangles from stl file (binary format).vi"("STL file path"=w321) -> ("Triangles array"=w327:T8[], "Error out"=w320:errorcluster)  [unwired: 1 out]
            n76 = call "Read triangles from stl file (binary format).vi"("STL file path"=w319) -> ("Triangles array"=w328:T8[], "Error out"=w316:errorcluster)  [unwired: 1 out]
            n77 = call "Read triangles from stl file (binary format).vi"("STL file path"=w313) -> ("Triangles array"=w307:T8[], "Error out"=w312:errorcluster)  [unwired: 1 out]
            n78 = call "Creat bounding sphere.vi"("Triangles"=w307) -> ("Bounding sphere"=w306:T9)
            n79 = Merge Errors(w311, w320, w316, w312) -> (w325:errorcluster)
            n80 = in-place {
              in-place-border: [w329] -> w304
              n81 = in-place-cluster #3(w306) -> ("Radius"=w331:sgl)
              n82 = global read "Collision Detection global.vi" "Traverse_XYZ look-out radius (model units)"() -> (w329:sgl)
              n83 = Add(x=w331, y=w329) -> (x+y=w330:sgl)
              n84 = in-place-cluster #3("Radius"=w330) -> (w305:T9)
            }
          }
        }
      }
      frame "Model rotation" {
        # "check if rotation axis coordinates have changed"
        # "check if rotation axis has changed (e.g from negation of angle)"
        # "check if rotation angle has changed"
        n85 = Subtract(x=w337, y=w334) -> (x-y=w336:sgl[])
        n86 = Subtract(x=w343, y=w344) -> (x-y=w368:sgl)
        n87 = Subtract(x=sgl 1.0, y=sgl 1.1920929e-07) -> (x-y=w338:sgl)
        n88 = call "Dot product.vi"("B"=w350, "A"=w345) -> ("A . B"=w349:sgl)
        n89 = call "Dot product.vi"("B"=w336, "A"=w336) -> ("A . B"=w340:sgl)
        n90 = Absolute Value(x=w368) -> (abs(x)=w376:sgl)
        n91 = Less?(x=w340, y=sgl 1.1920929e-07) -> (x < y?=w339:bool)
        n92 = Greater?(x=w349, y=w338) -> (0:w341:bool)
        n93 = Less?(x=w376, y=sgl 1.1920929e-07) -> (x < y?=w346:bool)
        n94 = And(x=w341, y=w339) -> (x .and. y?=w342:bool)
        n95 = case shown="False" w346 {
          tunnel: w369 -> [w389 w454]
          tunnel: w368 -> [w388 w453]
          tunnel: [w387 w452] -> w366
          tunnel: [w386 w451] -> w365
          tunnel: w364 -> [w385 w450]
          tunnel: [w384 w449] -> w361
          tunnel: w337 -> [w383 w448]
          tunnel: w350 -> [w382 w447]
          tunnel: w342 -> [w381 w446]
          tunnel: w344 -> [w380 w445]
          tunnel: w345 -> [w379 w444]
          tunnel: w343 -> [w378 w443]
          tunnel: w334 -> [w377 w442]
          frame False {
            n96 = case shown="True" w381 {
              tunnel: w382 -> [w396 w435]
              tunnel: w389 -> [w394 w436]
              tunnel: w388 -> [_ w425]
              tunnel: w383 -> [w395 w434]
              tunnel: [w393 w431] -> w387
              tunnel: [w392 w430] -> w386
              tunnel: [w391 w429] -> w384
              tunnel: w385 -> [_ _]
              tunnel: w380 -> [w399 _]
              tunnel: w379 -> [w398 _]
              tunnel: w378 -> [w397 _]
              tunnel: w377 -> [w390 _]
              frame False {
                # "rotation axis has changed."
                # "re-build octree, and update arrays"
                # "rotate back to original state, then rotate by new angle about new axis"
                n97 = Negate(x=w399) -> (-x=w405:sgl)
                n98 = Multiply(x=w397, y=sgl 3.1415927) -> (x*y=w403:sgl)
                n99 = Multiply(x=w405, y=sgl 3.1415927) -> (x*y=w407:sgl)
                n100 = Divide(x=w403, y=sgl 180.0) -> (x/y=w404:sgl)
                n101 = Divide(x=w407, y=sgl 180.0) -> (x/y=w406:sgl)
                n102 = for {
                  tunnel: w394 -> [w422] mode=indexing
                  tunnel: w398 -> [w421]
                  tunnel: w406 -> [w420]
                  tunnel: [w418] -> w400 mode=indexing
                  tunnel: w390 -> [w419]
                  workers-P: _ -> [_]
                  n103 = call "Rotate triangle about arbitrary axis.vi"("Rotation angle (rad)"=w420, "Rotation axis coordinates (x, y, z)"=w419, "Rotation axis (unit direction vector)\nanti-clockwise positive looking into axis"=w421, "Triangle in"=w422) -> ("Triangle out"=w418:T8)
                }
                n104 = for {
                  tunnel: w400 -> [w417] mode=indexing
                  tunnel: w396 -> [w416]
                  tunnel: w404 -> [w415]
                  tunnel: [w413] -> w393 mode=indexing
                  tunnel: w395 -> [w414]
                  workers-P: _ -> [_]
                  n105 = call "Rotate triangle about arbitrary axis.vi"("Rotation angle (rad)"=w415, "Rotation axis coordinates (x, y, z)"=w414, "Rotation axis (unit direction vector)\nanti-clockwise positive looking into axis"=w416, "Triangle in"=w417) -> ("Triangle out"=w413:T8)
                }
                n106 = global read "Collision Detection global.vi" "Model octree resolution (model units)"() -> (w410:sgl)
                n107 = call "Get World extent.vi"("Triangles"=w393) -> ("Pmax (x, y, z)"=w411:sgl[], "Pmin (x, y, z)"=w412:sgl[])
                n108 = call "Build Octree from triangles.vi"("Triangle array"=w393, "World Pmin (x, y, z)"=w412, "World Pmax (x, y, z)"=w411, "Octree resolution (model units)"=w410) -> ("Stack error"=w391:errorcluster, "Octree node array"=w392:T5[])  [unwired: 1 out]
              }
              frame True {
                # "rotation alone has changed. Incrementally rotate model triangles, re-build octree, and update arrays"
                n109 = Multiply(x=w425, y=sgl 3.1415927) -> (x*y=w424:sgl)
                n110 = Divide(x=w424, y=sgl 180.0) -> (x/y=w423:sgl)
                n111 = for {
                  tunnel: w436 -> [w441] mode=indexing
                  tunnel: w435 -> [w440]
                  tunnel: w423 -> [w439]
                  tunnel: [w437] -> w431 mode=indexing
                  tunnel: w434 -> [w438]
                  workers-P: _ -> [_]
                  n112 = call "Rotate triangle about arbitrary axis.vi"("Rotation angle (rad)"=w439, "Rotation axis coordinates (x, y, z)"=w438, "Rotation axis (unit direction vector)\nanti-clockwise positive looking into axis"=w440, "Triangle in"=w441) -> ("Triangle out"=w437:T8)
                }
                n113 = global read "Collision Detection global.vi" "Model octree resolution (model units)"() -> (w428:sgl)
                n114 = call "Get World extent.vi"("Triangles"=w431) -> ("Pmax (x, y, z)"=w432:sgl[], "Pmin (x, y, z)"=w433:sgl[])
                n115 = call "Build Octree from triangles.vi"("Triangle array"=w431, "World Pmin (x, y, z)"=w433, "World Pmax (x, y, z)"=w432, "Octree resolution (model units)"=w428) -> ("Stack error"=w429:errorcluster, "Octree node array"=w430:T5[])  [unwired: 1 out]
              }
            }
          }
          frame True {
            n116 = case shown="False" w446 {
              tunnel: w447 -> [w457 _]
              tunnel: w454 -> [w477 w488]
              tunnel: w453 -> [_ _]
              tunnel: w448 -> [w458 _]
              tunnel: [w456 w488] -> w452
              tunnel: [w474 w489] -> w451
              tunnel: [w473 errorcluster {"status"=FALSE, "code"=0, "source"=""} ("Stack error")] -> w449
              tunnel: w450 -> [_ w489]
              tunnel: w445 -> [w459 _]
              tunnel: w444 -> [w466 _]
              tunnel: w443 -> [w460 _]
              tunnel: w442 -> [w455 _]
              frame False {
                # "rotation axis has changed."
                # "re-build octree, and update arrays"
                # "rotate back to original state, then rotate by new angle about new axis"
                n117 = Negate(x=w459) -> (-x=w467:sgl)
                n118 = Multiply(x=w460, y=sgl 3.1415927) -> (x*y=w464:sgl)
                n119 = Multiply(x=w467, y=sgl 3.1415927) -> (x*y=w469:sgl)
                n120 = Divide(x=w464, y=sgl 180.0) -> (x/y=w465:sgl)
                n121 = Divide(x=w469, y=sgl 180.0) -> (x/y=w468:sgl)
                n122 = for {
                  tunnel: w477 -> [w487] mode=indexing
                  tunnel: w466 -> [w486]
                  tunnel: w468 -> [w485]
                  tunnel: [w483] -> w461 mode=indexing
                  tunnel: w455 -> [w484]
                  workers-P: _ -> [_]
                  n123 = call "Rotate triangle about arbitrary axis.vi"("Rotation angle (rad)"=w485, "Rotation axis coordinates (x, y, z)"=w484, "Rotation axis (unit direction vector)\nanti-clockwise positive looking into axis"=w486, "Triangle in"=w487) -> ("Triangle out"=w483:T8)
                }
                n124 = for {
                  tunnel: w461 -> [w482] mode=indexing
                  tunnel: w457 -> [w481]
                  tunnel: w465 -> [w480]
                  tunnel: [w478] -> w456 mode=indexing
                  tunnel: w458 -> [w479]
                  workers-P: _ -> [_]
                  n125 = call "Rotate triangle about arbitrary axis.vi"("Rotation angle (rad)"=w480, "Rotation axis coordinates (x, y, z)"=w479, "Rotation axis (unit direction vector)\nanti-clockwise positive looking into axis"=w481, "Triangle in"=w482) -> ("Triangle out"=w478:T8)
                }
                n126 = global read "Collision Detection global.vi" "Model octree resolution (model units)"() -> (w472:sgl)
                n127 = call "Get World extent.vi"("Triangles"=w456) -> ("Pmax (x, y, z)"=w475:sgl[], "Pmin (x, y, z)"=w476:sgl[])
                n128 = call "Build Octree from triangles.vi"("Triangle array"=w456, "World Pmin (x, y, z)"=w476, "World Pmax (x, y, z)"=w475, "Octree resolution (model units)"=w472) -> ("Stack error"=w473:errorcluster, "Octree node array"=w474:T5[])  [unwired: 1 out]
              }
              frame True {
                # "no change, continue as is"
              }
            }
          }
        }
        n129 = Merge Errors(w362, w361) -> (w363:errorcluster)
      }
      frame "Traverse translation" {
        # "extrusion mode. Convex hull.\nPut original traverse into 'swap' shift register, and swap back after all collision detection checks"
        # "omit sqrt for speed"
        # "check if position has changed"
        n130 = Subtract(x=w509, y=w539) -> (x-y=w533:sgl[])
        n131 = call "Dot product.vi"("B"=w533, "A"=w533) -> ("A . B"=w517:sgl)
        n132 = Less?(x=w517, y=sgl 1.1920929e-07) -> (x < y?=w537:bool)
        n133 = case shown="False" w537 {
          tunnel: w536 -> [w604 w617]
          tunnel: w535 -> [w598 w616]
          tunnel: w534 -> [w596 w615]
          tunnel: w533 -> [w591 _]
          tunnel: [w595 w617] -> w508
          tunnel: [w594 w616] -> w507
          tunnel: [w593 w615] -> w506
          tunnel: w513 -> [w592 w614]
          tunnel: [w590 w614] -> w512
          frame False {
            w600 = sgl 0.0 ("element")
            # "traverse has moved, translate triangles and update arrays as appropriate"
            n134 = Index Array(array=w591) -> (element=w603:sgl)  [unwired: 1 in]
            n135 = Index Array(array=w591) -> (element #1=w601:sgl, element #2=w602:sgl)  [unwired: 2 in]
            n136 = Build Array(w603, w600, w600) -> (w599:sgl[])
            n137 = Build Array(w601, w602, w600) -> (w597:sgl[])
            n138 = for {
              tunnel: w604 -> [w613] mode=indexing
              workers-P: _ -> [_]
              tunnel: w599 -> [w612]
              tunnel: [w611] -> w595 mode=indexing
              n139 = call "Translate triangle.vi"("Translation vector (dx, dy, dz)"=w612, "Triangle in"=w613) -> ("Triangle out"=w611:T8)
            }
            n140 = for {
              tunnel: w598 -> [w610] mode=indexing
              workers-P: _ -> [_]
              tunnel: w597 -> [w609]
              tunnel: [w608] -> w594 mode=indexing
              n141 = call "Translate triangle.vi"("Translation vector (dx, dy, dz)"=w609, "Triangle in"=w610) -> ("Triangle out"=w608:T8)
            }
            n142 = for {
              tunnel: w596 -> [w607] mode=indexing
              workers-P: _ -> [_]
              tunnel: w591 -> [w606]
              tunnel: [w605] -> w593 mode=indexing
              n143 = call "Translate triangle.vi"("Translation vector (dx, dy, dz)"=w606, "Triangle in"=w607) -> ("Triangle out"=w605:T8)
            }
            n144 = call "Translate sphere.vi"("Translation vector (dx, dy, dz)"=w591, "Sphere in"=w592) -> ("Sphere out"=w590:T9)
          }
          frame True {
            # "no change, continue as is"
          }
        }
        n145 = case shown="True" w511 {
          tunnel: w506 -> [w542 w555]
          tunnel: [w542 w547] -> w503
          tunnel: w509 -> [_ w574]
          tunnel: w510 -> [_ w575]
          tunnel: w507 -> [w543 w558]
          tunnel: w508 -> [w544 w562]
          tunnel: [w543 w546] -> w504
          tunnel: [w544 w552] -> w505
          tunnel: [w541 w562] -> w500
          tunnel: [w541 w558] -> w501
          tunnel: [w541 w555] -> w502
          tunnel: [w540 TRUE] -> w493
          tunnel: w492 -> [w540 _]
          frame False {
            w541 = T8[] [] ("Triangles array")
          }
          frame True {
            w573 = sgl 0.0 ("element")
            n146 = Subtract(x=w575, y=w574) -> (x-y=w569:sgl[])
            n147 = Index Array(array=w569) -> (element=w570:sgl)  [unwired: 1 in]
            n148 = Index Array(array=w569) -> (element #1=w572:sgl, element #2=w571:sgl)  [unwired: 2 in]
            n149 = Build Array(w570, w573, w573) -> (w567:sgl[])
            n150 = Build Array(w572, w571, w573) -> (w568:sgl[])
            n151 = for {
              tunnel: w562 -> [w578] mode=indexing
              workers-P: _ -> [_]
              tunnel: w567 -> [w577]
              tunnel: [w576] -> w563 mode=indexing
              n152 = call "Translate triangle.vi"("Translation vector (dx, dy, dz)"=w577, "Triangle in"=w578) -> ("Triangle out"=w576:T8)
            }
            n153 = for {
              tunnel: w558 -> [w581] mode=indexing
              workers-P: _ -> [_]
              tunnel: w568 -> [w580]
              tunnel: [w579] -> w560 mode=indexing
              n154 = call "Translate triangle.vi"("Translation vector (dx, dy, dz)"=w580, "Triangle in"=w581) -> ("Triangle out"=w579:T8)
            }
            n155 = for {
              tunnel: w555 -> [w584] mode=indexing
              workers-P: _ -> [_]
              tunnel: w569 -> [w583]
              tunnel: [w582] -> w557 mode=indexing
              n156 = call "Translate triangle.vi"("Translation vector (dx, dy, dz)"=w583, "Triangle in"=w584) -> ("Triangle out"=w582:T8)
            }
            n157 = Build Array (concatenate)(w562, w563) -> (w561:T8[])
            n158 = Build Array (concatenate)(w558, w560) -> (w559:T8[])
            n159 = Build Array (concatenate)(w555, w557) -> (w556:T8[])
            n160 = call "Triangles to vertices (without duplicates).vi"("Triangles"=w561) -> ("Vertices (without duplicates)"=w564:sgl[][])
            n161 = call "Triangles to vertices (without duplicates).vi"("Triangles"=w559) -> ("Vertices (without duplicates)"=w565:sgl[][])
            n162 = call "Triangles to vertices (without duplicates).vi"("Triangles"=w556) -> ("Vertices (without duplicates)"=w566:sgl[][])
            n163 = call "Convex Hull 3D (GiftWrap).vi"("Vertices"=w564) -> ("Convex hull triangles, indexed"=w554:T10[])  [unwired: 1 out]
            n164 = call "Convex Hull 3D (GiftWrap).vi"("Vertices"=w565) -> ("Convex hull triangles, indexed"=w551:T10[])  [unwired: 1 out]
            n165 = call "Convex Hull 3D (GiftWrap).vi"("Vertices"=w566) -> ("Convex hull triangles, indexed"=w550:T10[])  [unwired: 1 out]
            n166 = call "Adapt triangles.vi"("Triangles in (indexed type)"=w554) -> ("Triangles out (full type)"=w553:T8[])
            n167 = call "Adapt triangles.vi"("Triangles in (indexed type)"=w551) -> ("Triangles out (full type)"=w549:T8[])
            n168 = call "Adapt triangles.vi"("Triangles in (indexed type)"=w550) -> ("Triangles out (full type)"=w548:T8[])
            n169 = call "Process adapted triangles (full).vi"("Triangles in"=w553) -> ("Triangles out"=w552:T8[])
            n170 = call "Process adapted triangles (full).vi"("Triangles in"=w549) -> ("Triangles out"=w546:T8[])
            n171 = call "Process adapted triangles (full).vi"("Triangles in"=w548) -> ("Triangles out"=w547:T8[])
          }
        }
        n172 = case shown="\"Traverse - All\", Default" w515 {
          tunnel: ["Collision detection: Traverse - Tunnel" "Collision detection: Traverse - Model" "Collision detection: Traverse - Fixed objects" "Collision detection: Traverse - Traverse" "Collision detection: Traverse - Tunnel"] -> w514
          frame "Traverse - Tunnel" {
          }
          frame "Traverse - Model" {
          }
          frame "Traverse - Fixed objects" {
          }
          frame "Traverse - Traverse" {
          }
          frame "Traverse - All", Default {
          }
        }
        n173 = Select(t="Render graphics", s=w524, f="End") -> (s? t:f=w522:string)
        n174 = Select(t=w522, s=w526, f=w514) -> (s? t:f=w525:string)
      }
      frame "Collision detection: Traverse - Tunnel" {
        # "Distinguish traverse part involved in collision"
        # "Only work with desired parts of traverse. Note XYZ is always checked(!)"
        # "If desired, and no collision, perform minimum separation test within sphere of influence"
        # "Checks traverse triangles against tunnel octree (and then triangles if necessary)"
        n175 = case shown="\"X and XY and XYZ\"" w632 {
          tunnel: w663 -> [_ w685]
          tunnel: [sgl[][] [] ("Collision point(s)") w683] -> w650
          tunnel: [i32[] [] ("Indices of possible triangles") w682] -> w649
          tunnel: w639 -> [_ w681]
          tunnel: w638 -> [_ w680]
          tunnel: [FALSE w679] -> w624
          frame Default {
          }
          frame "X and XY and XYZ" {
            n176 = for {
              workers-P: _ -> [_]
              tunnel: w685 -> [w693] mode=indexing
              tunnel: w680 -> [w692]
              tunnel: w681 -> [w691]
              tunnel: [w689] -> w684 mode=indexing
              tunnel: [w690] -> w683 mode=concatenating if=w689
              tunnel: [w687] -> w682 mode=concatenating if=w686
              n177 = call "Collision test simple.vi"("Octree for query triangles"=w691, "Query triangles"=w692, "Triangle to test"=w693) -> ("Indices of possible triangles"=w687:i32[], "Collision point(s)"=w690:sgl[][], "Collision(s)?"=w689:bool)
              n178 = Empty Array?(array=w687) -> (empty?=w688:bool)
              n179 = Not(x=w688) -> (.not. x?=w686:bool)
            }
            n180 = Or Array Elements(Boolean array=w684) -> (logical OR=w679:bool)
          }
        }
        n181 = case shown="\"XY and XYZ\", \"X and XY and XYZ\"" w632 {
          tunnel: w662 -> [_ w703]
          tunnel: [sgl[][] [] ("Collision point(s)") w701] -> w652
          tunnel: [i32[] [] ("Indices of possible triangles") w700] -> w648
          tunnel: w639 -> [_ w699]
          tunnel: w638 -> [_ w698]
          tunnel: [FALSE w697] -> w623
          frame Default {
          }
          frame "XY and XYZ", "X and XY and XYZ" {
            n182 = for {
              workers-P: _ -> [_]
              tunnel: w703 -> [w711] mode=indexing
              tunnel: w698 -> [w710]
              tunnel: w699 -> [w709]
              tunnel: [w707] -> w702 mode=indexing
              tunnel: [w708] -> w701 mode=concatenating if=w707
              tunnel: [w705] -> w700 mode=concatenating if=w704
              n183 = call "Collision test simple.vi"("Octree for query triangles"=w709, "Query triangles"=w710, "Triangle to test"=w711) -> ("Indices of possible triangles"=w705:i32[], "Collision point(s)"=w708:sgl[][], "Collision(s)?"=w707:bool)
              n184 = Empty Array?(array=w705) -> (empty?=w706:bool)
              n185 = Not(x=w706) -> (.not. x?=w704:bool)
            }
            n186 = Or Array Elements(Boolean array=w702) -> (logical OR=w697:bool)
          }
        }
        n187 = for {
          workers-P: _ -> [_]
          tunnel: w640 -> [w675] mode=indexing
          tunnel: w638 -> [w674]
          tunnel: w639 -> [w673]
          tunnel: [w671] -> w631 mode=indexing
          tunnel: [w672] -> w651 mode=concatenating if=w671
          tunnel: [w669] -> w647 mode=concatenating if=w668
          n188 = call "Collision test simple.vi"("Octree for query triangles"=w673, "Query triangles"=w674, "Triangle to test"=w675) -> ("Indices of possible triangles"=w669:i32[], "Collision point(s)"=w672:sgl[][], "Collision(s)?"=w671:bool)
          n189 = Empty Array?(array=w669) -> (empty?=w670:bool)
          n190 = Not(x=w670) -> (.not. x?=w668:bool)
        }
        n191 = Or Array Elements(Boolean array=w631) -> (logical OR=w622:bool)
        n192 = Bundle(cluster=cluster{"X":bool, "XY":bool, "XYZ":bool} {"X"=FALSE, "XY"=FALSE, "XYZ"=FALSE} ("Traverse collision part"), "X"=w624, "XY"=w623, "XYZ"=w622) -> (w621:cluster{"X":bool, "XY":bool, "XYZ":bool})
        n193 = Compound Arithmetic op=OR(w624, w623, w622) -> (w633:bool)
        n194 = Build Array (concatenate)(w649, w648, w647) -> (w646:i32[])
        n195 = call "Remove duplicate indices.vi"("I32 array with duplicates"=w646) -> ("I32 array without duplicates"=w642:i32[])
        n196 = case shown="True" w633 {
          selector: w633 -> [w722 w724]
          tunnel: w652 -> [_ w728]
          tunnel: w651 -> [_ w727]
          tunnel: w650 -> [_ w726]
          tunnel: [sgl[][] [] w725] -> w656
          tunnel: [w722 w724] -> w645
          frame False {
          }
          frame True {
            n197 = Build Array (concatenate)(w726, w728, w727) -> (w725:sgl[][])
          }
        }
        n198 = Compound Arithmetic op=AND(invert w645, w644) -> (w643:bool)
        n199 = case shown="True" w643 {
          tunnel: [sgl 0.0 ("Minimum separation") w720] -> w659
          tunnel: [sgl[] [] ("Minimum separation vector\n(from all test triangles)") w721] -> w658
          tunnel: w642 -> [w714 _]
          tunnel: [w714 w719] -> w641
          tunnel: w640 -> [_ w718]
          tunnel: w637 -> [_ w717]
          tunnel: w639 -> [_ w716]
          tunnel: w638 -> [_ w715]
          frame False {
          }
          frame True {
            n200 = call "Get minimum separation within sphere.vi"("Triangles to test"=w718, "Query triangles"=w715, "Octree for query triangles"=w716, "Sphere of interest"=w717) -> ("Minimum separation vector\n(from all test triangles)"=w721:sgl[], "Minimum separation"=w720:sgl, "Indices of possible triangles"=w719:i32[])  [unwired: 2 in]
          }
        }
        n201 = case shown="\"Traverse - All\"" w655 {
          tunnel: w654 -> [_ w731]
          tunnel: ["Collision detection: Traverse - Model" w730] -> w653
          frame "Traverse - All" {
          }
          frame Default {
            n202 = Select(t="Render graphics", s=w731, f="End") -> (s? t:f=w730:string)
          }
        }
      }
      frame "Collision detection: Traverse - Model" {
        # "Distinguish traverse part involved in collision"
        # "Only work with desired parts of traverse. Note XYZ is always checked(!)"
        # "append to existing values in case of \"all\" collision mode"
        # "Checks traverse triangles against model octree (and then triangles if necessary)"
        n203 = case shown="\"X and XY and XYZ\"" w758 {
          tunnel: w796 -> [w825 _]
          tunnel: [w823 sgl[][] [] ("Collision point(s)")] -> w779
          tunnel: [w822 i32[] [] ("Indices of possible triangles")] -> w776
          tunnel: w752 -> [w821 _]
          tunnel: w766 -> [w820 _]
          tunnel: [w819 FALSE] -> w739
          frame "X and XY and XYZ" {
            n204 = for {
              workers-P: _ -> [_]
              tunnel: w825 -> [w833] mode=indexing
              tunnel: w821 -> [w832]
              tunnel: w820 -> [w831]
              tunnel: [w829] -> w824 mode=indexing
              tunnel: [w830] -> w823 mode=concatenating if=w829
              tunnel: [w827] -> w822 mode=concatenating if=w826
              n205 = call "Collision test simple.vi"("Octree for query triangles"=w831, "Query triangles"=w832, "Triangle to test"=w833) -> ("Indices of possible triangles"=w827:i32[], "Collision point(s)"=w830:sgl[][], "Collision(s)?"=w829:bool)
              n206 = Empty Array?(array=w827) -> (empty?=w828:bool)
              n207 = Not(x=w828) -> (.not. x?=w826:bool)
            }
            n208 = Or Array Elements(Boolean array=w824) -> (logical OR=w819:bool)
          }
          frame Default {
          }
        }
        n209 = case shown="\"XY and XYZ\", \"X and XY and XYZ\"" w758 {
          tunnel: w793 -> [_ w810]
          tunnel: [sgl[][] [] ("Collision point(s)") w808] -> w778
          tunnel: [i32[] [] ("Indices of possible triangles") w807] -> w775
          tunnel: w752 -> [_ w806]
          tunnel: w766 -> [_ w805]
          tunnel: [FALSE w804] -> w738
          frame Default {
          }
          frame "XY and XYZ", "X and XY and XYZ" {
            n210 = for {
              workers-P: _ -> [_]
              tunnel: w810 -> [w818] mode=indexing
              tunnel: w806 -> [w817]
              tunnel: w805 -> [w816]
              tunnel: [w814] -> w809 mode=indexing
              tunnel: [w815] -> w808 mode=concatenating if=w814
              tunnel: [w812] -> w807 mode=concatenating if=w811
              n211 = call "Collision test simple.vi"("Octree for query triangles"=w816, "Query triangles"=w817, "Triangle to test"=w818) -> ("Indices of possible triangles"=w812:i32[], "Collision point(s)"=w815:sgl[][], "Collision(s)?"=w814:bool)
              n212 = Empty Array?(array=w812) -> (empty?=w813:bool)
              n213 = Not(x=w813) -> (.not. x?=w811:bool)
            }
            n214 = Or Array Elements(Boolean array=w809) -> (logical OR=w804:bool)
          }
        }
        n215 = for {
          workers-P: _ -> [_]
          tunnel: w767 -> [w867] mode=indexing
          tunnel: w752 -> [w866]
          tunnel: w766 -> [w865]
          tunnel: [w863] -> w780 mode=indexing
          tunnel: [w864] -> w777 mode=concatenating if=w863
          tunnel: [w861] -> w774 mode=concatenating if=w860
          n216 = call "Collision test simple.vi"("Octree for query triangles"=w865, "Query triangles"=w866, "Triangle to test"=w867) -> ("Indices of possible triangles"=w861:i32[], "Collision point(s)"=w864:sgl[][], "Collision(s)?"=w863:bool)
          n217 = Empty Array?(array=w861) -> (empty?=w862:bool)
          n218 = Not(x=w862) -> (.not. x?=w860:bool)
        }
        n219 = Or Array Elements(Boolean array=w780) -> (logical OR=w737:bool)
        n220 = Unbundle(w746) -> ("X"=w743:bool, "XY"=w744:bool, "XYZ"=w745:bool)
        n221 = Or(x=w737, y=w745) -> (x .or. y?=w740:bool)
        n222 = Or(x=w738, y=w744) -> (x .or. y?=w741:bool)
        n223 = Compound Arithmetic op=OR(w739, w738, w737) -> (w759:bool)
        n224 = Build Array (concatenate)(w776, w775, w774) -> (w773:i32[])
        n225 = Or(x=w739, y=w743) -> (x .or. y?=w742:bool)
        n226 = Bundle(cluster=w746, "X"=w742, "XY"=w741, "XYZ"=w740) -> (w736:cluster{"X":bool, "XY":bool, "XYZ":bool})
        n227 = case shown="True" w759 {
          selector: w759 -> [w854 w855]
          tunnel: w779 -> [_ w859]
          tunnel: w778 -> [_ w858]
          tunnel: w777 -> [_ w857]
          tunnel: [sgl[][] [] w856] -> w781
          tunnel: [w854 w855] -> w783
          frame False {
          }
          frame True {
            n228 = Build Array (concatenate)(w859, w858, w857) -> (w856:sgl[][])
          }
        }
        n229 = call "Remove duplicate indices.vi"("I32 array with duplicates"=w773) -> ("I32 array without duplicates"=w769:i32[])
        n230 = Or(x=w783, y=w782) -> (x .or. y?=w768:bool)
        n231 = Empty Array?(array=w752) -> (empty?=w749:bool)
        n232 = Compound Arithmetic op=AND(invert w749, invert w768, w765) -> (w772:bool)
        n233 = case shown="True" w772 {
          tunnel: [w839 w851] -> w770
          tunnel: [w840 w852] -> w771
          tunnel: w769 -> [w842 _]
          tunnel: [w842 w850] -> w753
          tunnel: w767 -> [_ w849]
          tunnel: w764 -> [_ w848]
          tunnel: w766 -> [_ w847]
          tunnel: w752 -> [_ w846]
          tunnel: w751 -> [w838 _]
          tunnel: w750 -> [w841 _]
          tunnel: w749 -> [w837 _]
          frame False {
            n234 = case shown="True" w837 {
              tunnel: w841 -> [_ w845]
              tunnel: [_ w845] -> w840
              tunnel: [sgl 0.0 ("Minimum separation") w844] -> w839
              tunnel: w838 -> [_ w844]
              frame False {
              }
              frame True {
              }
            }
          }
          frame True {
            n235 = call "Get minimum separation within sphere.vi"("Triangles to test"=w849, "Query triangles"=w846, "Octree for query triangles"=w847, "Sphere of interest"=w848) -> ("Minimum separation vector\n(from all test triangles)"=w852:sgl[], "Minimum separation"=w851:sgl, "Indices of possible triangles"=w850:i32[])  [unwired: 2 in]
          }
        }
        n236 = Less?(x=w770, y=w751) -> (x < y?=w789:bool)
        n237 = case shown="True" w789 {
          tunnel: w751 -> [w873 _]
          tunnel: w770 -> [_ w875]
          tunnel: [w873 w875] -> w788
          tunnel: w771 -> [_ w876]
          tunnel: [w874 w876] -> w787
          tunnel: w750 -> [w874 _]
          frame False {
          }
          frame True {
          }
        }
        n238 = Build Array (concatenate)(w760, w781) -> (w790:sgl[][])
        n239 = case shown="\"Traverse - All\"" w786 {
          tunnel: w784 -> [_ w870]
          tunnel: ["Collision detection: Traverse - Fixed objects" w869] -> w785
          frame "Traverse - All" {
          }
          frame Default {
            n240 = Select(t="Render graphics", s=w870, f="End") -> (s? t:f=w869:string)
          }
        }
      }
      frame "Collision detection: Traverse - Fixed objects" {
        # "Distinguish traverse part involved in collision"
        # "Only work with desired parts of traverse. Note XYZ is always checked(!)"
        # "append to existing values in case of \"all\" collision mode"
        # "Checks traverse triangles against fixed objects octree (and then triangles if necessary)"
        n241 = case shown="\"X and XY and XYZ\"" w901 {
          tunnel: w940 -> [w969 _]
          tunnel: [w967 sgl[][] [] ("Collision point(s)")] -> w923
          tunnel: [w966 i32[] [] ("Indices of possible triangles")] -> w920
          tunnel: w895 -> [w965 _]
          tunnel: w898 -> [w964 _]
          tunnel: [w963 FALSE] -> w881
          frame "X and XY and XYZ" {
            n242 = for {
              workers-P: _ -> [_]
              tunnel: w969 -> [w977] mode=indexing
              tunnel: w965 -> [w976]
              tunnel: w964 -> [w975]
              tunnel: [w973] -> w968 mode=indexing
              tunnel: [w974] -> w967 mode=concatenating if=w973
              tunnel: [w971] -> w966 mode=concatenating if=w970
              n243 = call "Collision test simple.vi"("Octree for query triangles"=w975, "Query triangles"=w976, "Triangle to test"=w977) -> ("Indices of possible triangles"=w971:i32[], "Collision point(s)"=w974:sgl[][], "Collision(s)?"=w973:bool)
              n244 = Empty Array?(array=w971) -> (empty?=w972:bool)
              n245 = Not(x=w972) -> (.not. x?=w970:bool)
            }
            n246 = Or Array Elements(Boolean array=w968) -> (logical OR=w963:bool)
          }
          frame Default {
          }
        }
        n247 = case shown="\"XY and XYZ\", \"X and XY and XYZ\"" w901 {
          tunnel: w937 -> [_ w954]
          tunnel: [sgl[][] [] ("Collision point(s)") w952] -> w922
          tunnel: [i32[] [] ("Indices of possible triangles") w951] -> w919
          tunnel: w895 -> [_ w950]
          tunnel: w898 -> [_ w949]
          tunnel: [FALSE w948] -> w880
          frame Default {
          }
          frame "XY and XYZ", "X and XY and XYZ" {
            n248 = for {
              workers-P: _ -> [_]
              tunnel: w954 -> [w962] mode=indexing
              tunnel: w950 -> [w961]
              tunnel: w949 -> [w960]
              tunnel: [w958] -> w953 mode=indexing
              tunnel: [w959] -> w952 mode=concatenating if=w958
              tunnel: [w956] -> w951 mode=concatenating if=w955
              n249 = call "Collision test simple.vi"("Octree for query triangles"=w960, "Query triangles"=w961, "Triangle to test"=w962) -> ("Indices of possible triangles"=w956:i32[], "Collision point(s)"=w959:sgl[][], "Collision(s)?"=w958:bool)
              n250 = Empty Array?(array=w956) -> (empty?=w957:bool)
              n251 = Not(x=w957) -> (.not. x?=w955:bool)
            }
            n252 = Or Array Elements(Boolean array=w953) -> (logical OR=w948:bool)
          }
        }
        n253 = for {
          workers-P: _ -> [_]
          tunnel: w911 -> [w1011] mode=indexing
          tunnel: w895 -> [w1010]
          tunnel: w898 -> [w1009]
          tunnel: [w1007] -> w924 mode=indexing
          tunnel: [w1008] -> w921 mode=concatenating if=w1007
          tunnel: [w1005] -> w918 mode=concatenating if=w1004
          n254 = call "Collision test simple.vi"("Octree for query triangles"=w1009, "Query triangles"=w1010, "Triangle to test"=w1011) -> ("Indices of possible triangles"=w1005:i32[], "Collision point(s)"=w1008:sgl[][], "Collision(s)?"=w1007:bool)
          n255 = Empty Array?(array=w1005) -> (empty?=w1006:bool)
          n256 = Not(x=w1006) -> (.not. x?=w1004:bool)
        }
        n257 = Or Array Elements(Boolean array=w924) -> (logical OR=w879:bool)
        n258 = Unbundle(w883) -> ("X"=w887:bool, "XY"=w888:bool, "XYZ"=w889:bool)
        n259 = Or(x=w879, y=w889) -> (x .or. y?=w884:bool)
        n260 = Or(x=w880, y=w888) -> (x .or. y?=w885:bool)
        n261 = Compound Arithmetic op=OR(w881, w880, w879) -> (w902:bool)
        n262 = Build Array (concatenate)(w920, w919, w918) -> (w917:i32[])
        n263 = Or(x=w881, y=w887) -> (x .or. y?=w886:bool)
        n264 = Bundle(cluster=w883, "X"=w886, "XY"=w885, "XYZ"=w884) -> (w882:cluster{"X":bool, "XY":bool, "XYZ":bool})
        n265 = case shown="True" w902 {
          selector: w902 -> [w998 w999]
          tunnel: w923 -> [_ w1003]
          tunnel: w922 -> [_ w1002]
          tunnel: w921 -> [_ w1001]
          tunnel: [sgl[][] [] w1000] -> w925
          tunnel: [w998 w999] -> w927
          frame False {
          }
          frame True {
            n266 = Build Array (concatenate)(w1003, w1002, w1001) -> (w1000:sgl[][])
          }
        }
        n267 = call "Remove duplicate indices.vi"("I32 array with duplicates"=w917) -> ("I32 array without duplicates"=w913:i32[])
        n268 = Or(x=w927, y=w926) -> (x .or. y?=w912:bool)
        n269 = Empty Array?(array=w895) -> (empty?=w892:bool)
        n270 = Compound Arithmetic op=AND(invert w892, invert w912, w908) -> (w916:bool)
        n271 = case shown="True" w916 {
          tunnel: [w984 w995] -> w914
          tunnel: [w982 w996] -> w915
          tunnel: w913 -> [w986 _]
          tunnel: [w986 w994] -> w897
          tunnel: w911 -> [_ w993]
          tunnel: w907 -> [_ w992]
          tunnel: w898 -> [_ w991]
          tunnel: w895 -> [_ w990]
          tunnel: w894 -> [w983 _]
          tunnel: w893 -> [w985 _]
          tunnel: w892 -> [w981 _]
          frame False {
            n272 = case shown="True" w981 {
              tunnel: [sgl 0.0 ("Minimum separation") w989] -> w984
              tunnel: w985 -> [_ w989]
              tunnel: w983 -> [_ w988]
              tunnel: [_ w988] -> w982
              frame False {
              }
              frame True {
              }
            }
          }
          frame True {
            n273 = call "Get minimum separation within sphere.vi"("Triangles to test"=w993, "Query triangles"=w990, "Octree for query triangles"=w991, "Sphere of interest"=w992) -> ("Minimum separation vector\n(from all test triangles)"=w996:sgl[], "Minimum separation"=w995:sgl, "Indices of possible triangles"=w994:i32[])  [unwired: 2 in]
          }
        }
        n274 = Less?(x=w914, y=w893) -> (x < y?=w933:bool)
        n275 = case shown="True" w933 {
          tunnel: w893 -> [w1017 _]
          tunnel: w914 -> [_ w1019]
          tunnel: [w1017 w1019] -> w932
          tunnel: w915 -> [_ w1020]
          tunnel: [w1018 w1020] -> w931
          tunnel: w894 -> [w1018 _]
          frame False {
          }
          frame True {
          }
        }
        n276 = Build Array (concatenate)(w903, w925) -> (w934:sgl[][])
        n277 = case shown="\"Traverse - All\"" w930 {
          tunnel: w928 -> [_ w1014]
          tunnel: ["Collision detection: Traverse - Traverse" w1013] -> w929
          frame "Traverse - All" {
          }
          frame Default {
            n278 = Select(t="Render graphics", s=w1014, f="End") -> (s? t:f=w1013:string)
          }
        }
      }
      frame "Collision detection: Traverse - Traverse" {
        # "NOT YET IMPLEMENTED!"
        n279 = Select(t="Render graphics", s=w1052, f="End") -> (s? t:f=w1051:string)
      }
      frame "Render graphics" {
        w1083 = T4 {"Red"=0.66, "Green"=0.5, "Blue"=0.5, "Alpha"=1.0} ("Colour")
        w1073 = T4 {"Red"=0.25, "Green"=0.25, "Blue"=0.25, "Alpha"=1.0} ("Colour")
        w1070 = T11."Polygons" ("Render mode")
        n280 = Empty Array?(array=w1104) -> (empty?=w1103:bool)
        n281 = Not(x=w1103) -> (.not. x?=w1102:bool)
        n282 = global read "Collision Detection global.vi" "Draw octree leaf-node boxes"() -> (w1090:bool)
        n283 = global read "Collision Detection global.vi" "Highlight tested triangles"() -> (w1066:bool)
        n284 = And(x=w1102, y=w1066) -> (x .and. y?=w1101:bool)
        n285 = case shown="True" w1101 {
          tunnel: w1129 -> [w1203 w1215]
          tunnel: T4 {"Red"=1.0, "Green"=1.0, "Blue"=1.0, "Alpha"=1.0} ("Colour") -> [w1202 w1216]
          tunnel: w1070 -> [w1201 w1211]
          tunnel: [w1200 w1205] -> w1120
          tunnel: [w1198 w1210] -> w1105
          tunnel: w1104 -> [_ w1214]
          frame False {
            n286 = call "Create triangles mesh.vi"("Colour"=w1202, "Render mode"=w1201, "Triangles array"=w1203) -> ("Error out"=w1200:errorcluster, "Triangle mesh out"=w1199:refnum<vi>)
            n287 = Build Array(w1199) -> (w1198:refnum<vi>[])
          }
          frame True {
            n288 = for {
              tunnel: w1215 -> [w1225] mode=indexing
              tunnel: w1214 -> [w1223]
              tunnel: [w1225] -> w1213 mode=indexing if=w1220
              tunnel: [w1225] -> w1212 mode=indexing if=w1224
              shift-right: [w1218] -> _
              shift-left: 0 -> [w1219]
              i -> [w1221]
              n289 = Index Array(array=w1223, index=w1219) -> (element=w1222:i32)
              n290 = Equal?(x=w1222, y=w1221) -> (x = y?=w1220:bool)
              n291 = case shown="True" w1220 {
                tunnel: w1219 -> [w1226 w1228]
                tunnel: [w1226 w1227] -> w1218
                frame False {
                }
                frame True {
                  n292 = Increment(x=w1228) -> (x+1=w1227:i32)
                }
              }
              n293 = Not(x=w1220) -> (.not. x?=w1224:bool)
            }
            n294 = call "Create triangles mesh.vi"("Colour"=w1216, "Render mode"=w1211, "Triangles array"=w1212) -> ("Error out"=w1207:errorcluster, "Triangle mesh out"=w1209:refnum<vi>)
            n295 = call "Create triangles mesh.vi"("Colour"=T4 {"Red"=0.75, "Green"=1.0, "Blue"=1.0, "Alpha"=1.0}, "Render mode"=w1211, "Triangles array"=w1213) -> ("Error out"=w1206:errorcluster, "Triangle mesh out"=w1208:refnum<vi>)
            n296 = Build Array(w1209, w1208) -> (w1210:refnum<vi>[])
            n297 = Merge Errors(w1207, w1206) -> (w1205:errorcluster)
          }
        }
        n298 = Empty Array?(array=w1064) -> (empty?=w1099:bool)
        n299 = Not(x=w1099) -> (.not. x?=w1100:bool)
        n300 = And(x=w1100, y=w1066) -> (x .and. y?=w1085:bool)
        n301 = case shown="True" w1085 {
          tunnel: w1087 -> [w1172 w1184]
          tunnel: w1073 -> [w1171 w1185]
          tunnel: w1070 -> [w1170 w1180]
          tunnel: [w1169 w1174] -> w1084
          tunnel: [w1167 w1179] -> w1086
          tunnel: w1064 -> [_ w1183]
          frame False {
            n302 = call "Create triangles mesh.vi"("Colour"=w1171, "Render mode"=w1170, "Triangles array"=w1172) -> ("Error out"=w1169:errorcluster, "Triangle mesh out"=w1168:refnum<vi>)
            n303 = Build Array(w1168) -> (w1167:refnum<vi>[])
          }
          frame True {
            n304 = for {
              tunnel: w1184 -> [w1194] mode=indexing
              tunnel: w1183 -> [w1192]
              tunnel: [w1194] -> w1182 mode=indexing if=w1189
              tunnel: [w1194] -> w1181 mode=indexing if=w1193
              shift-right: [w1187] -> _
              shift-left: 0 -> [w1188]
              i -> [w1190]
              n305 = Index Array(array=w1192, index=w1188) -> (element=w1191:i32)
              n306 = Equal?(x=w1191, y=w1190) -> (x = y?=w1189:bool)
              n307 = case shown="True" w1189 {
                tunnel: w1188 -> [w1195 w1197]
                tunnel: [w1195 w1196] -> w1187
                frame False {
                }
                frame True {
                  n308 = Increment(x=w1197) -> (x+1=w1196:i32)
                }
              }
              n309 = Not(x=w1189) -> (.not. x?=w1193:bool)
            }
            n310 = call "Create triangles mesh.vi"("Colour"=w1185, "Render mode"=w1180, "Triangles array"=w1181) -> ("Error out"=w1176:errorcluster, "Triangle mesh out"=w1178:refnum<vi>)
            n311 = call "Create triangles mesh.vi"("Colour"=T4 {"Red"=1.0, "Green"=0.85, "Blue"=0.0, "Alpha"=1.0}, "Render mode"=w1180, "Triangles array"=w1182) -> ("Error out"=w1175:errorcluster, "Triangle mesh out"=w1177:refnum<vi>)
            n312 = Build Array(w1178, w1177) -> (w1179:refnum<vi>[])
            n313 = Merge Errors(w1176, w1175) -> (w1174:errorcluster)
          }
        }
        n314 = Empty Array?(array=w1063) -> (empty?=w1068:bool)
        n315 = Not(x=w1068) -> (.not. x?=w1067:bool)
        n316 = And(x=w1067, y=w1066) -> (x .and. y?=w1065:bool)
        n317 = case shown="True" w1065 {
          tunnel: w1071 -> [w1141 w1153]
          tunnel: w1073 -> [w1140 w1154]
          tunnel: w1070 -> [w1139 w1149]
          tunnel: [w1138 w1143] -> w1069
          tunnel: [w1136 w1148] -> w1072
          tunnel: w1063 -> [_ w1152]
          frame False {
            n318 = call "Create triangles mesh.vi"("Colour"=w1140, "Render mode"=w1139, "Triangles array"=w1141) -> ("Error out"=w1138:errorcluster, "Triangle mesh out"=w1137:refnum<vi>)
            n319 = Build Array(w1137) -> (w1136:refnum<vi>[])
          }
          frame True {
            n320 = for {
              tunnel: w1153 -> [w1163] mode=indexing
              tunnel: w1152 -> [w1161]
              tunnel: [w1163] -> w1151 mode=indexing if=w1158
              tunnel: [w1163] -> w1150 mode=indexing if=w1162
              shift-right: [w1156] -> _
              shift-left: 0 -> [w1157]
              i -> [w1159]
              n321 = Index Array(array=w1161, index=w1157) -> (element=w1160:i32)
              n322 = Equal?(x=w1160, y=w1159) -> (x = y?=w1158:bool)
              n323 = case shown="True" w1158 {
                tunnel: w1157 -> [w1164 w1166]
                tunnel: [w1164 w1165] -> w1156
                frame False {
                }
                frame True {
                  n324 = Increment(x=w1166) -> (x+1=w1165:i32)
                }
              }
              n325 = Not(x=w1158) -> (.not. x?=w1162:bool)
            }
            n326 = call "Create triangles mesh.vi"("Colour"=w1154, "Render mode"=w1149, "Triangles array"=w1150) -> ("Error out"=w1145:errorcluster, "Triangle mesh out"=w1147:refnum<vi>)
            n327 = call "Create triangles mesh.vi"("Colour"=T4 {"Red"=1.0, "Green"=0.85, "Blue"=0.0, "Alpha"=1.0}, "Render mode"=w1149, "Triangles array"=w1151) -> ("Error out"=w1144:errorcluster, "Triangle mesh out"=w1146:refnum<vi>)
            n328 = Build Array(w1147, w1146) -> (w1148:refnum<vi>[])
            n329 = Merge Errors(w1145, w1144) -> (w1143:errorcluster)
          }
        }
        n330 = call "Create triangles mesh.vi"("Colour"=w1083, "Render mode"=w1070, "Triangles array"=w1128) -> ("Error out"=w1119:errorcluster, "Triangle mesh out"=w1111:refnum<vi>)
        n331 = call "Create triangles mesh.vi"("Colour"=w1083, "Render mode"=w1070, "Triangles array"=w1127) -> ("Error out"=w1118:errorcluster, "Triangle mesh out"=w1110:refnum<vi>)
        n332 = call "Create triangles mesh.vi"("Colour"=w1083, "Render mode"=w1070, "Triangles array"=w1126) -> ("Error out"=w1117:errorcluster, "Triangle mesh out"=w1109:refnum<vi>)
        n333 = Build Array (concatenate)(w1105, w1086, w1072, w1111, w1110, w1109) -> (w1097:refnum<vi>[])
        n334 = case shown="True" w1090 {
          tunnel: w1125 -> [_ w1253]
          tunnel: w1124 -> [_ w1252]
          tunnel: T4 {"Red"=0.0, "Green"=0.25, "Blue"=0.0, "Alpha"=1.0} ("Colour (emission)") -> [_ w1249]
          tunnel: T4 {"Red"=0.0, "Green"=0.5, "Blue"=0.5, "Alpha"=1.0} ("Colour (emission)") -> [_ w1248]
          tunnel: [errorcluster {"status"=FALSE, "code"=0, "source"=""} ("error IO") w1242] -> w1116
          tunnel: [w1240 w1241] -> w1096
          tunnel: w1097 -> [w1240 w1245]
          frame False {
          }
          frame True {
            n335 = call "Create Octree node boxes.vi"("Colour (emission)"=w1249, "Draw populated leaf nodes only"=TRUE, "Octree nodes array"=w1253) -> ("Error out"=w1244:errorcluster, "Octree node boxes array"=w1247:refnum<vi>[])
            n336 = call "Create Octree node boxes.vi"("Colour (emission)"=w1248, "Draw populated leaf nodes only"=TRUE, "Octree nodes array"=w1252) -> ("Error out"=w1243:errorcluster, "Octree node boxes array"=w1246:refnum<vi>[])
            n337 = Build Array (concatenate)(w1245, w1247, w1246) -> (w1241:refnum<vi>[])
            n338 = Merge Errors(w1244, w1243) -> (w1242:errorcluster)
          }
        }
        n339 = global read "Collision Detection global.vi" "Collision marker radius (mm)"() -> (w1089:sgl)
        n340 = Empty Array?(array=w1062) -> (empty?=w1106:bool)
        n341 = case shown="False" w1106 {
          tunnel: T3 {"Red"=1.0, "Green"=0.0, "Blue"=0.0, "Alpha"=1.0} ("Colour") -> [w1236 _]
          tunnel: w1089 -> [w1235 _]
          tunnel: w1070 -> [w1234 _]
          tunnel: [w1233 errorcluster {"status"=FALSE, "code"=0, "source"=""} ("error IO")] -> w1115
          tunnel: [w1231 w1238] -> w1095
          tunnel: w1096 -> [w1232 w1238]
          tunnel: w1062 -> [w1229 _]
          frame False {
            n342 = call "Create spheres.vi"("Render mode"=w1234, "Colour"=w1236, "Radius (model units)"=w1235, "Points array"=w1229) -> ("Error out"=w1233:errorcluster, "Points"=w1230:refnum<vi>[])
            n343 = Build Array (concatenate)(w1232, w1230) -> (w1231:refnum<vi>[])
          }
          frame True {
          }
        }
        n344 = global read "Collision Detection global.vi" "Camera Position"() -> (w1093:T12)
        n345 = global read "Collision Detection global.vi" "Reset camera"() -> (w1082:bool)
        n346 = global read "Collision Detection global.vi" "Up Direction"() -> (w1091:T12)
        n347 = global read "Collision Detection global.vi" "Target"() -> (w1092:T12)
        n348 = call "Create new scene.vi"("Translation"=cluster{"X":sgl, "Y":sgl, "Z":sgl} {"X"=0.0, "Y"=0.0, "Z"=0.0}, "Scale"=cluster{"X":sgl, "Y":sgl, "Z":sgl} {"X"=1.0, "Y"=1.0, "Z"=1.0}, "Scene objects array"=w1095) -> ("Error out"=w1114:errorcluster, "Scene out"=w1098:refnum<vi>)
        n349 = call "3D display.vi"("Camera Position"=w1093, "Scene in"=w1098, "Target"=w1092, "Up Direction"=w1091, "Reset camera"=w1082) -> ()  [unwired: 1 in]
        n350 = Merge Errors(w1113, w1120, w1084, w1069, w1119, w1118, w1117, w1116, w1115, w1114) -> (w1112:errorcluster)
      }
      frame "End" {
        # "Min. sep. dist. is returned as -1 if the option is enabled and no objects were detected within sphere radius.\nNaN is returned if the option is disabled (can use this rather than check the boolean)."
        n351 = case shown="True" w1255 {
          tunnel: w1258 -> [_ w1296]
          tunnel: w1257 -> [_ w1293]
          tunnel: [sgl nan ("t") w1292] -> w1256
          frame False {
          }
          frame True {
            n352 = Empty Array?(array=w1296) -> (empty?=w1295:bool)
            n353 = Select(t=sgl -1.0, s=w1295, f=w1293) -> (s? t:f=w1292:sgl)
          }
        }
        n354 = case shown="True" w1278 {
          tunnel: w1277 -> [_ w1304]
          tunnel: w1276 -> [_ w1303]
          tunnel: w1275 -> [_ w1302]
          tunnel: [w1300 w1304] -> w1274
          tunnel: [w1299 w1303] -> w1273
          tunnel: [w1298 w1302] -> w1272
          tunnel: w1271 -> [w1298 _]
          tunnel: w1270 -> [w1299 _]
          tunnel: w1269 -> [w1300 _]
          tunnel: [w1297 FALSE] -> w1260
          tunnel: w1259 -> [w1297 _]
          frame False {
          }
          frame True {
          }
        }
      }
    }
  }
  "Collision" <- w20
  "Minimum separation" <- w19
  "Minimum separation vector (from trav.)" <- w18
  "Collision point(s)" <- w17
  "Error out" <- w16
  "Traverse collision part" <- w2
